vi "Main.vi"(11 "Module Admin":refnum<class "Delacor_lib_QMH_Module Admin.lvclass">) -> ()   [LabVIEW 2019, in "Acquisition.lvlib"]
doc: "This template is based off of the Queued Message Handler design pattern and the Queued Message Handler project template that ships with LabVIEW.\n\nThe main difference is that the queue is private to this module and communication between modules is performed via Broadcast and Request events.\n\nRequest events are wrapped in public API methods and are handled in the Event Handling Loop (EHL) of this VI. Any module can register for Broadcast events sent by this module. The EHL generates messages based on user interface actions.\n\nThe Message Handling Loop (MHL) processes messages generated by the EHL, or by other messages. The messages are string values, so new messages can be added easily to the Message Cases case structure in the MHL. Each message cluster can also provide an optional value for Message Data, which is a variant that can be converted to whatever message-specific data is required.\n_____\nBased on Delacor QMH Project Template 4.0.0.47.\n_____\nBased on DQMH Project Template 6.1.0.94.\n\n<b>Note:</b> This VI was modified by the <b>Validate DQMH Module</b> tool to add a 'Panel Hidden' status updated broadcast to the Panel Close? event when External Launch = TRUE.\n\n<b>Note:</b> This VI was modified by the <b>Validate DQMH Module</b> tool to add a call to the Error Reported VI at the end of the 'Exit' MHL frame."
uses:
  Acquisition.lvlib
  <vilib>/Delacor/Delacor QMH/Libraries/Module Admin_class/Delacor_lib_QMH_Module Admin.lvclass
  Module Data--cluster.ctl
  Signal Type--enum.ctl
  Calibration Values--cluster.ctl
  WiBCI16T_Data.ctl
  WiBCI16T_Status.ctl
  Reg_Map.ctl
  Acquisition Types.ctl
  Stop Argument--cluster.ctl
  <vilib>/Delacor/Delacor QMH/Libraries/Message Queue_class/Delacor_lib_QMH_Message Queue.lvclass/Delacor_lib_QMH_Message Queue.ctl
  <vilib>/Delacor/Delacor QMH/Libraries/Module Admin_class/Delacor_lib_QMH_Module Admin.lvclass/Delacor_lib_QMH_Module Admin.ctl
  Start Acquiring Argument--cluster.ctl
  Start Acquiring (Reply Payload)--cluster.ctl
  Stop Acquiring Argument--cluster.ctl
  Settings Editor/Update Application Settings (Reply Payload)--cluster.ctl
  Settings Editor/Settings--cluster.ctl
  CML Shared/EEG Channel Settings.ctl
  Command_TestData Argument--cluster.ctl
  Check WiFi AP Argument--cluster.ctl
  Command_NoiseData Argument--cluster.ctl
  Command_LiveData Argument--cluster.ctl
  Command_ImpedanceData Argument--cluster.ctl
  Command_GoToIdle Argument--cluster.ctl
  Soft Trigger Argument--cluster.ctl
  Start IMP Acquiring Argument--cluster.ctl
  Stop IMP acquiring Argument--cluster.ctl
  Start GND Loop acquiring Argument--cluster.ctl
  Start CNV Acquiring Argument--cluster.ctl
  Start EOC Acquiring Argument--cluster.ctl
  Command_GndImpedanceData Argument--cluster.ctl
  <vilib>/Utility/miscctls.llb/LVPointTypeDef.ctl
  <vilib>/Delacor/Delacor QMH/Libraries/Message Queue_class/Delacor_lib_QMH_Enqueue Message (Single).vi
  <vilib>/Delacor/Delacor QMH/Libraries/Module Admin_class/Delacor_lib_QMH_Get External Launch.vi
  <userlib>/_MGI/1D Array/MGI Calculate Array Differences/MGI Calculate Array Differences (DBL[]).vi
  <userlib>/_MGI/Timing/MGI Wait/MGI Wait (U32).vi
  <vilib>/Utility/error.llb/Error Cluster From Error Code.vi
  <vilib>/ErrorRing/Error Ring.xnode
  <vilib>/Delacor/Delacor QMH/Libraries/Message Queue_class/Delacor_lib_QMH_Message Queue.lvclass
  Settings Editor/Settings Editor.lvlib
  Logger/Logger.lvlib
  CML UI/CML UI.lvlib
  CML Shared/CML Shared.lvlib
  Lab Streaming Layer/Lab Streaming Layer.lvlib
panel:
  out "Settings":T1 {"WiBCI16T Data"."Reg Map"."ADS2" format="%x"; "WiBCI16T Data"."Reg Map"."ADS1" format="%x"}
  out "error out":errorcluster
  # "This is a headless module. Show its panel to confirm that the Settings are updated correctly and other debugging tasks. Use the Settings Editor to change the settings for this module."
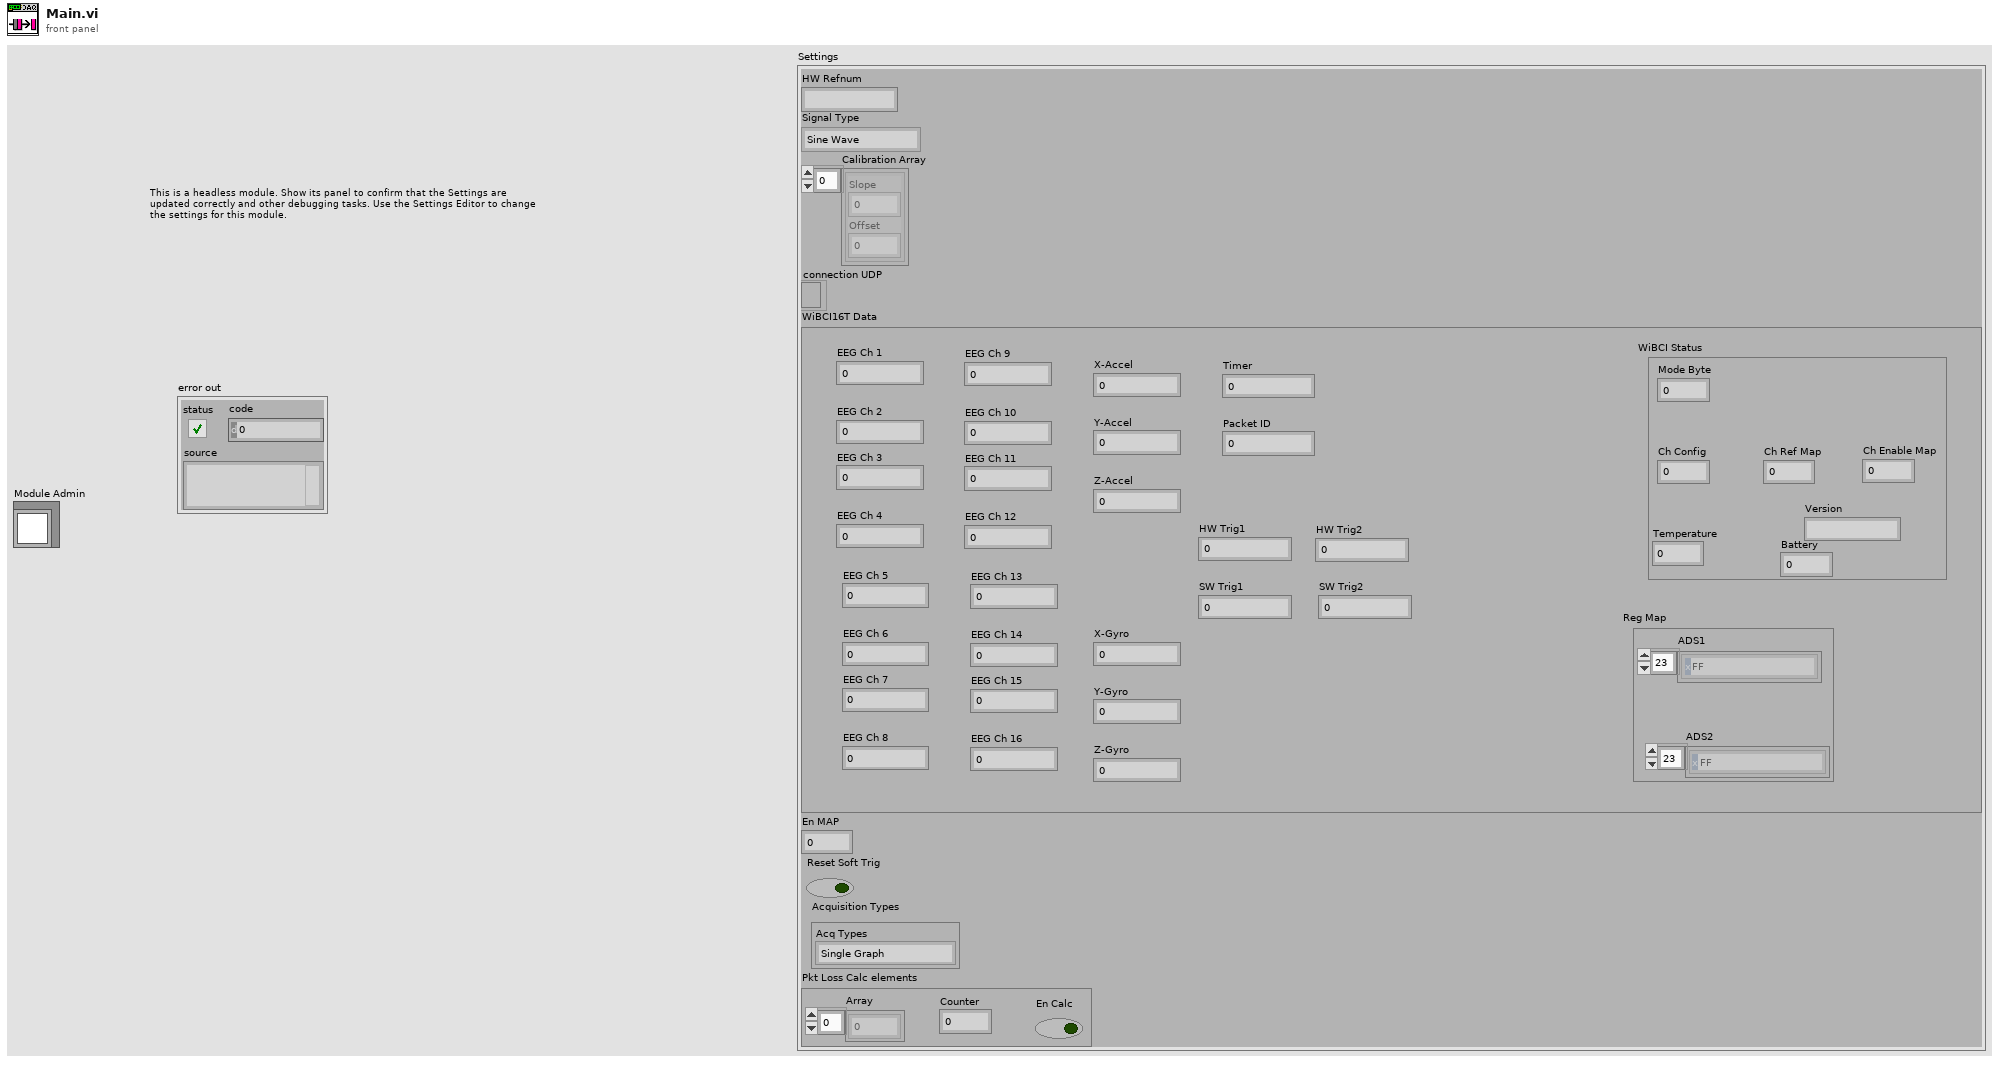
[diagram p1: front panel]
types:
  T1 = typedef "Acquisition.lvlib/Module Data--cluster.ctl" = cluster{"HW Refnum":string, "Signal Type":T2, "Calibration Array":T3[], "connection UDP":refnum<k16>, "WiBCI16T Data":T4, "En MAP":u16, "Reset Soft Trig":bool, "Acquisition Types":T7, "Pkt Loss Calc elements":cluster{"Array":u32[], "Counter":u32, "En Calc":bool}}
  T2 = typedef "Acquisition.lvlib/Signal Type--enum.ctl" = enum16{"Sine Wave", "Square with Noise"}
  T3 = typedef "Acquisition.lvlib/Calibration Values--cluster.ctl" = cluster{"Slope":dbl, "Offset":dbl}
  T4 = typedef "Acquisition.lvlib/WiBCI16T_Data.ctl" = cluster{"EEG Ch 1":dbl, "EEG Ch 2":dbl, "EEG Ch 3":dbl, "EEG Ch 4":dbl, "EEG Ch 5":dbl, "EEG Ch 6":dbl, "EEG Ch 7":dbl, "EEG Ch 8":dbl, "EEG Ch 9":dbl, "EEG Ch 10":dbl, "EEG Ch 11":dbl, "EEG Ch 12":dbl, "EEG Ch 13":dbl, "EEG Ch 14":dbl, "EEG Ch 15":dbl, "EEG Ch 16":dbl, "X-Accel":i16, "Y-Accel":i16, "Z-Accel":i16, "X-Gyro":i16, "Y-Gyro":i16, "Z-Gyro":i16, "Timer":u32, "Packet ID":u32, "HW Trig1":u8, "SW Trig1":i8, "HW Trig2":u8, "SW Trig2":i8, "WiBCI Status":T5, "Reg Map":T6}
  T5 = typedef "Acquisition.lvlib/WiBCI16T_Status.ctl" = cluster{"Mode Byte":u8, "Ch Config":u8, "Ch Ref Map":u16, "Ch Enable Map":u16, "Temperature":sgl, "Battery":u8, "Version":string}
  T6 = typedef "Acquisition.lvlib/Reg_Map.ctl" = cluster{"ADS1":u8[], "ADS2":u8[]}
  T7 = typedef "Acquisition.lvlib/Acquisition Types.ctl" = cluster{"Acq Types":enum16{"Single Graph", "Eyes O/C", "CNV Demo", "Impedance", "Graph"}}
  T8 = typedef "Settings Editor.lvlib/Broadcast Events--cluster.ctl" = cluster{"Module Did Init":refnum<user-event>, "Status Updated":refnum<user-event>, "Error Reported":refnum<user-event>, "Module Did Stop":refnum<user-event>, "Update Module Execution Status":refnum<user-event>, "Application Settings Updated":refnum<user-event>}
  T9 = typedef "Acquisition.lvlib/Request Events--cluster.ctl" = cluster{"Stop Module":refnum<user-event>, "Show Panel":refnum<user-event>, "Hide Panel":refnum<user-event>, "Get Module Execution Status":refnum<user-event>, "Show Diagram":refnum<user-event>, "Stop Acquiring":refnum<user-event>, "Wakeup Helper Loop":refnum<user-event>, "Change Settings":refnum<user-event>, "Calibrate DAQ":refnum<user-event>, "Start Acquiring":refnum<user-event>, "Command_TestData":refnum<user-event>, "Check WiFi AP":refnum<user-event>, "Command_NoiseData":refnum<user-event>, "Command_LiveData":refnum<user-event>, "Command_ImpedanceData":refnum<user-event>, "Command_GoToIdle":refnum<user-event>, "Soft Trigger":refnum<user-event>, "Start IMP Acquiring":refnum<user-event>, "Stop IMP acquiring":refnum<user-event>, "Start GND Loop acquiring":refnum<user-event>, "IMP data updated":refnum<user-event>, "Start CNV Acquiring":refnum<user-event>, "Start EOC Acquiring":refnum<user-event>, "Private":cluster{"Wake-up Helper Loop for Pkt Loss Calc":refnum<user-event>, "Stop Pkt Loss Calc":refnum<user-event>, "Update Packet ID":refnum<user-event>, "Calculate Packet Loss":refnum<user-event>}, "Command_GndImpedanceData":refnum<user-event>}
  T10 = enum32{"invalid lock state", "Not Locked", "Locked (No Password)", "Password-protected"}
  T11 = typedef "Acquisition.lvlib/Stop Argument--cluster.ctl" = cluster{"Origin":string, "Exit via Stop Module Req?":bool, "Wait for Module to stop?":bool}
  T12 = typedef "Acquisition.lvlib/Start Acquiring Argument--cluster.ctl" = cluster{"Wait Notifier":refnum<notifier>, "wait for reply":bool}
  T13 = typedef "Acquisition.lvlib/Stop Acquiring Argument--cluster.ctl" = cluster{"Boolean":bool}
  T14 = typedef "Settings Editor.lvlib/Update Application Settings (Reply Payload)--cluster.ctl" = cluster{"Settings":T15, "error":errorcluster}
  T15 = typedef "Settings Editor.lvlib/Settings--cluster.ctl" = cluster{"Signal Type":T2, "Calibration Array":T3[], "Log File Base Path":path, "EEG Channels":T16, "Soft Trig enum":enum16{"Disable Soft Trigger", "Enable Soft Trigger"}, "Montage selection":cluster{"Montages Ref":refnum<vi>, "Selected Montage Number":u8, "Montages Names":string[]}, "LSL En enum":enum16{"LSL Disabled", "LSL Enabled"}}
  T16 = typedef "CML Shared.lvlib/EEG Channel Settings.ctl" = cluster{"16 EEG Channels":cluster{"Channel Name":string, "Channel No":u8, "Channel Enabled":bool, "Channel Referenced":bool}[], "Gain":u8}
  T17 = typedef "Acquisition.lvlib/Command_TestData Argument--cluster.ctl" = cluster{"Boolean":bool}
  T18 = typedef "Acquisition.lvlib/Check WiFi AP Argument--cluster.ctl" = cluster{"Connected ?":bool}
  T19 = typedef "Acquisition.lvlib/Command_NoiseData Argument--cluster.ctl" = cluster{"Boolean":bool}
  T20 = typedef "Acquisition.lvlib/Command_LiveData Argument--cluster.ctl" = cluster{"Boolean":bool}
  T21 = typedef "Acquisition.lvlib/Command_ImpedanceData Argument--cluster.ctl" = cluster{"Boolean":bool}
  T22 = typedef "Acquisition.lvlib/Command_GoToIdle Argument--cluster.ctl" = cluster{"Boolean":bool}
  T23 = typedef "Acquisition.lvlib/Soft Trigger Argument--cluster.ctl" = cluster{"Value":i8}
  T24 = typedef "Acquisition.lvlib/Start IMP Acquiring Argument--cluster.ctl" = cluster{"Boolean":bool}
  T25 = typedef "Acquisition.lvlib/Stop IMP acquiring Argument--cluster.ctl" = cluster{"Boolean":bool}
  T26 = typedef "Acquisition.lvlib/Start GND Loop acquiring Argument--cluster.ctl" = cluster{"Boolean":bool}
  T27 = typedef "Acquisition.lvlib/Start CNV Acquiring Argument--cluster.ctl" = cluster{"Boolean":bool}
  T28 = typedef "Acquisition.lvlib/Start EOC Acquiring Argument--cluster.ctl" = cluster{"Boolean":bool}
  T29 = typedef "Acquisition.lvlib/Command_GndImpedanceData Argument--cluster.ctl" = cluster{"Boolean":bool}
  T30 = typedef "LVPointTypeDef.ctl" = cluster{"Horizontal":i16, "Vertical":i16}
  T31 = enum32{"Invalid", "Standard", "Closed", "Hidden", "Minimized", "Maximized"}
  T32 = enum16{"Single Graph", "Eyes O/C", "CNV Demo", "Impedance", "Graph"}
  T33 = typedef "Acquisition.lvlib/Start Acquiring (Reply Payload)--cluster.ctl" = cluster{"HW ID":string, "error":errorcluster, "UDP connection ID ":refnum<k16>}
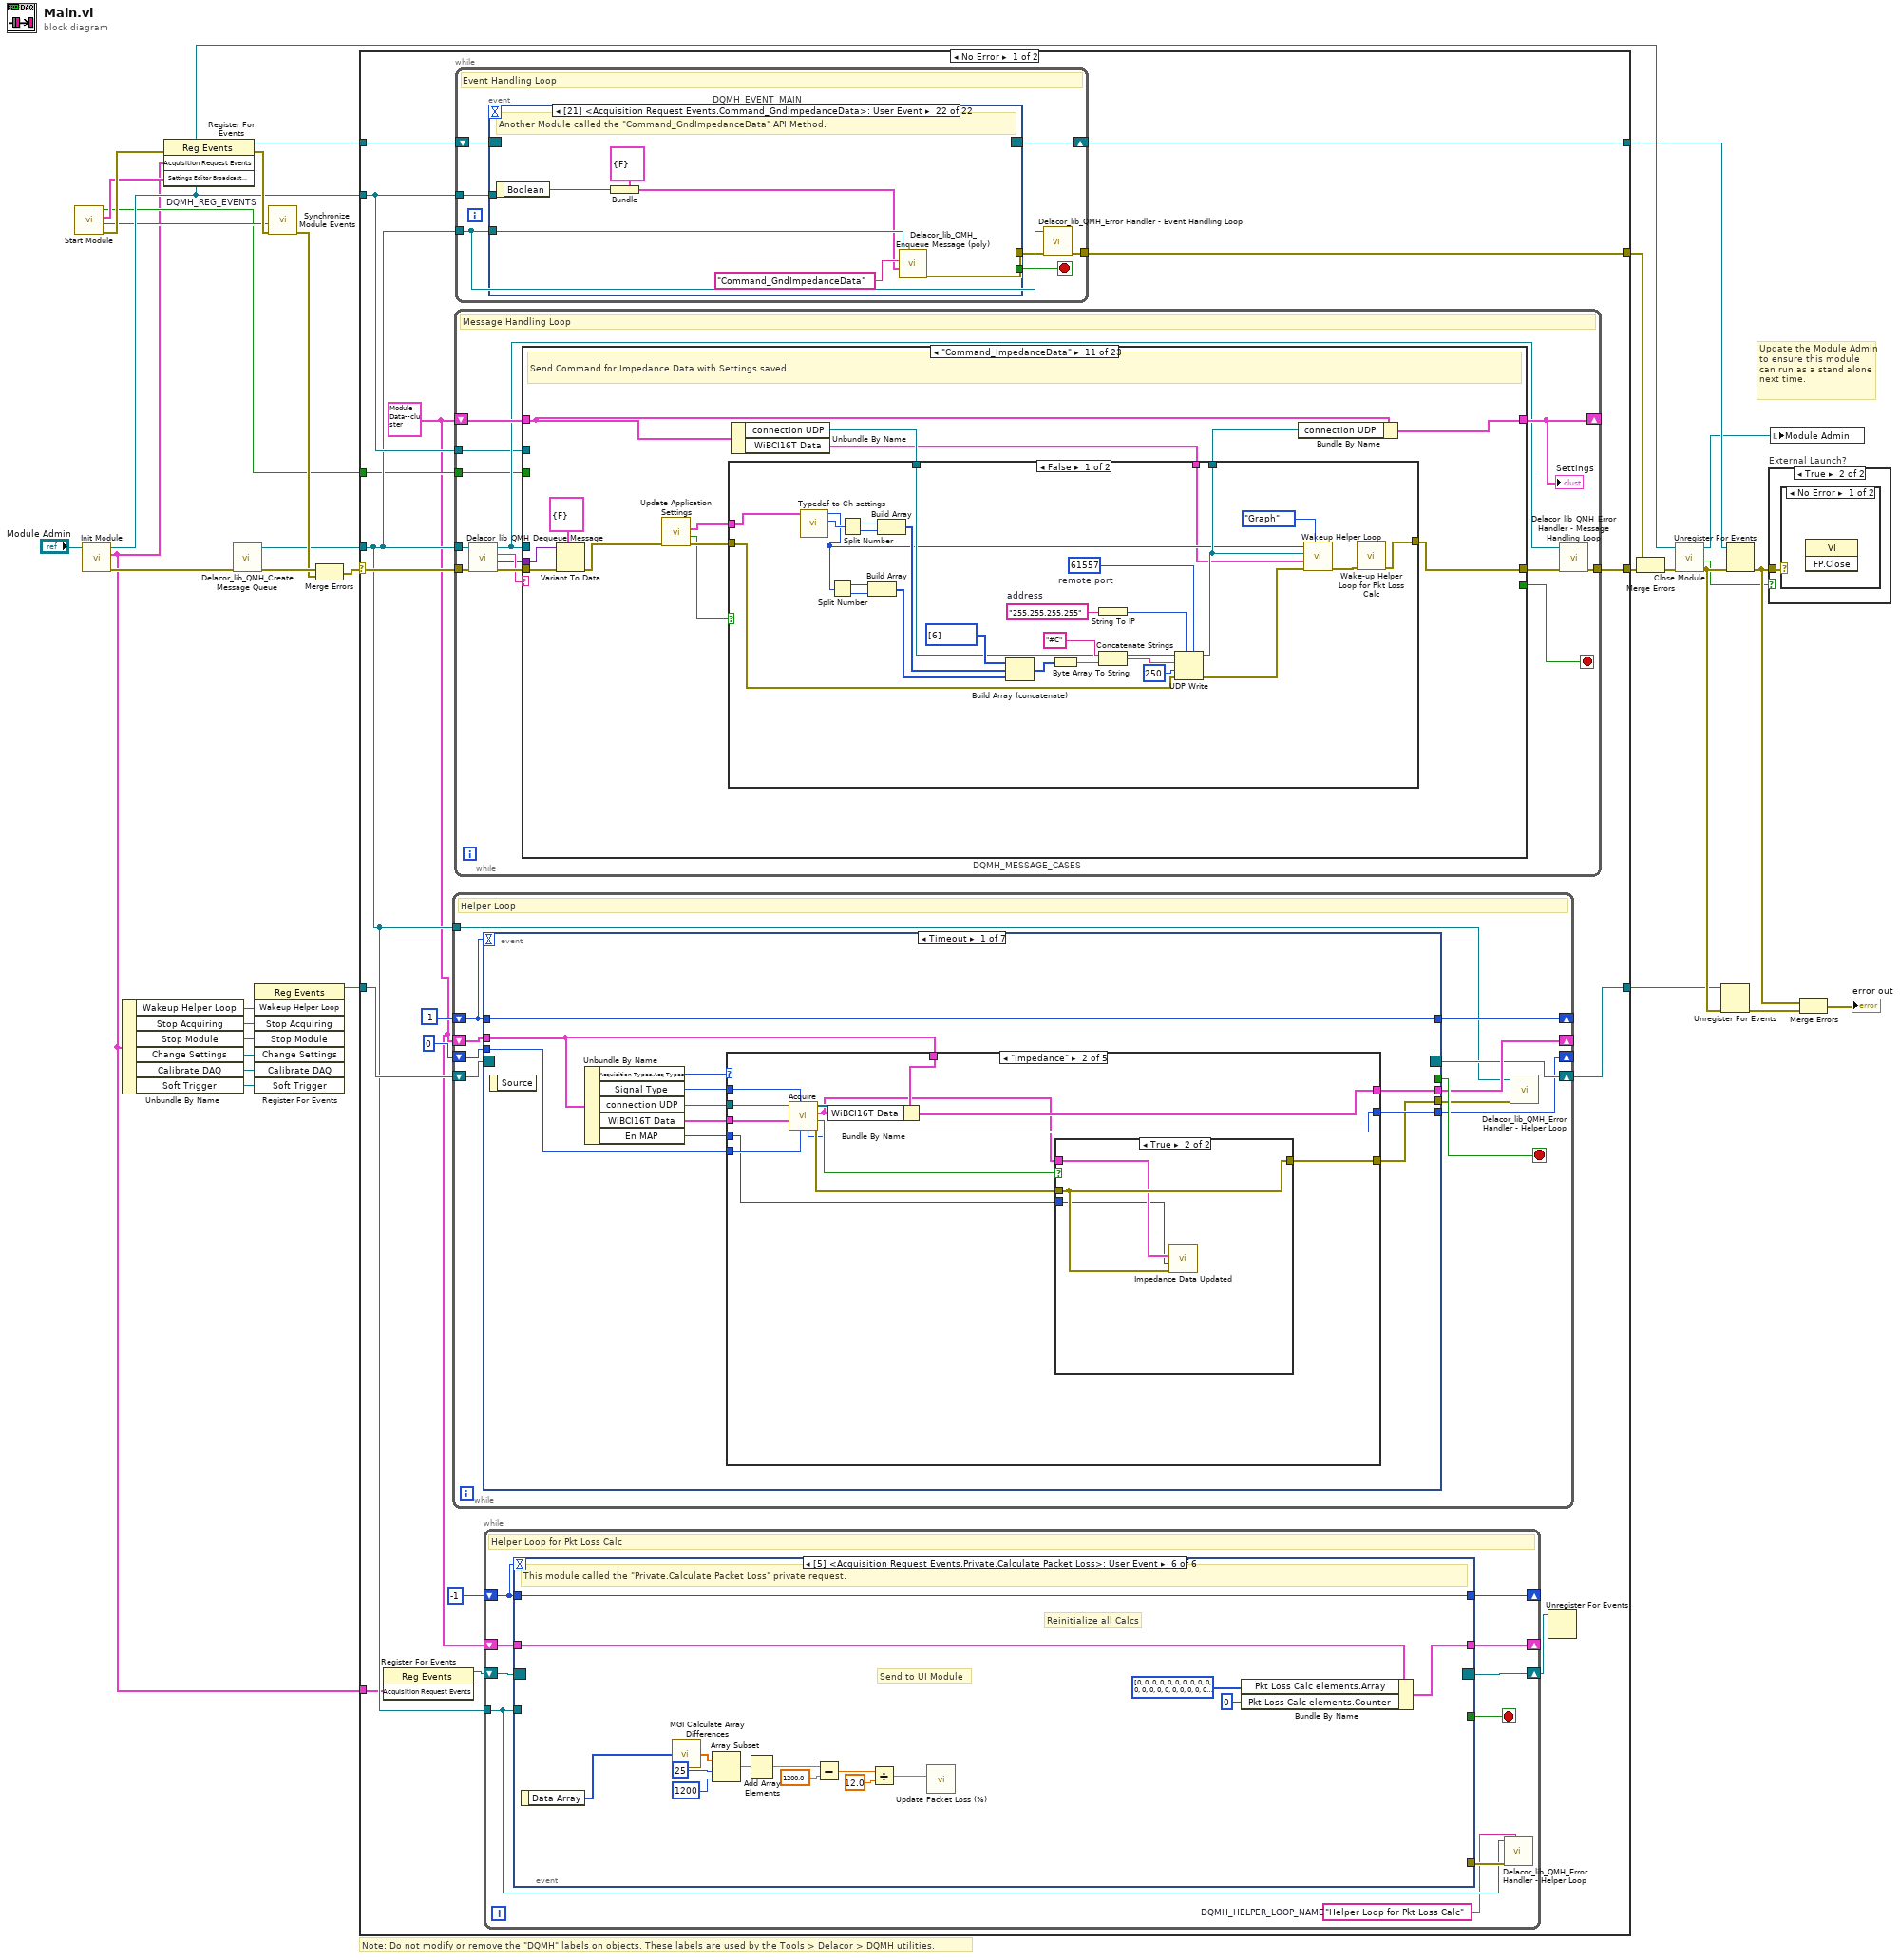
[diagram p0: block diagram]
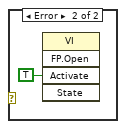
[diagram p3: hidden frame]
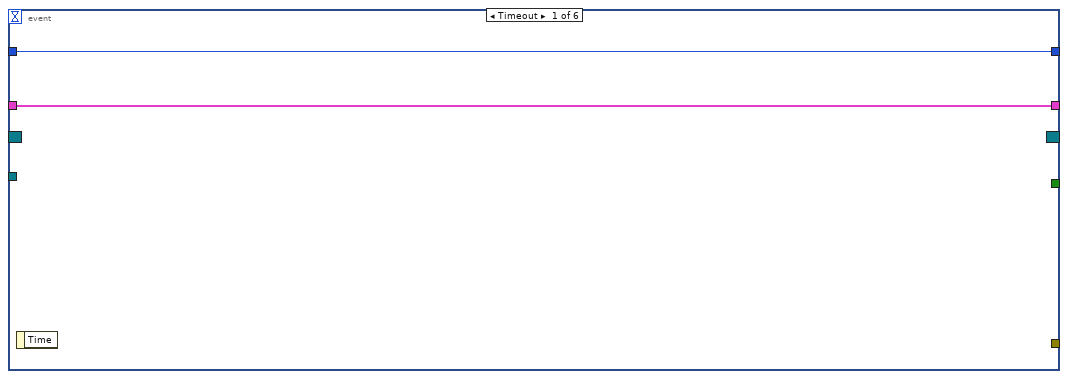
[diagram p4: hidden frame]
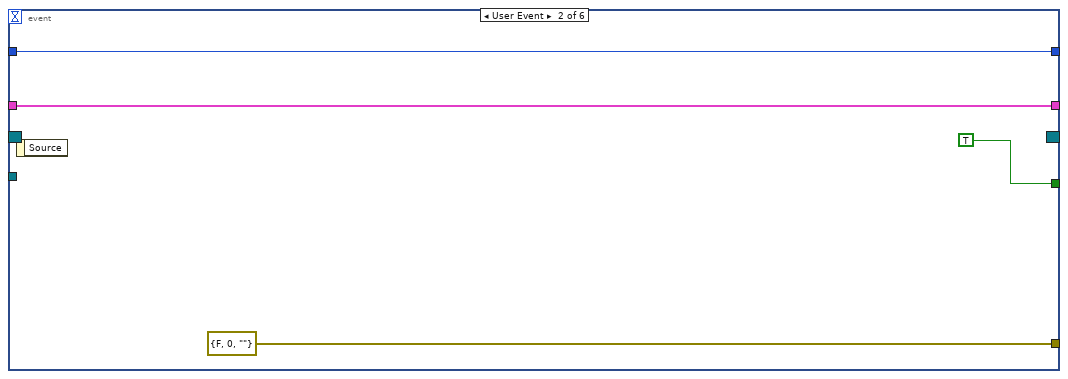
[diagram p5: hidden frame]
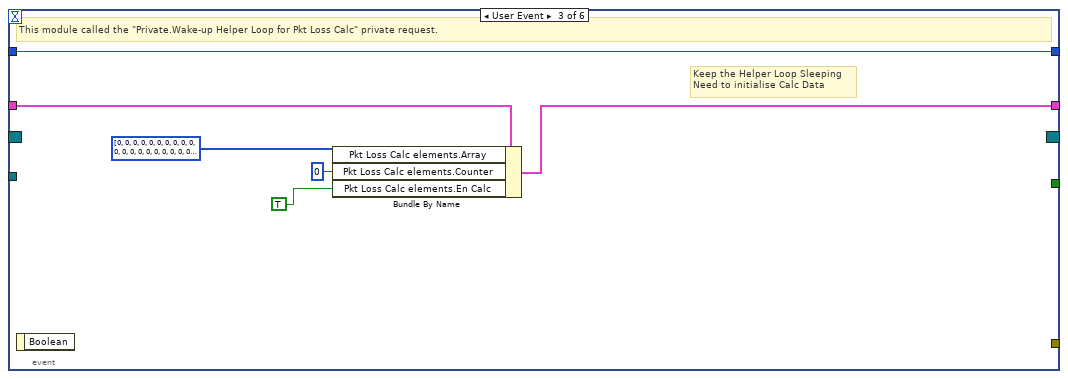
[diagram p6: hidden frame]
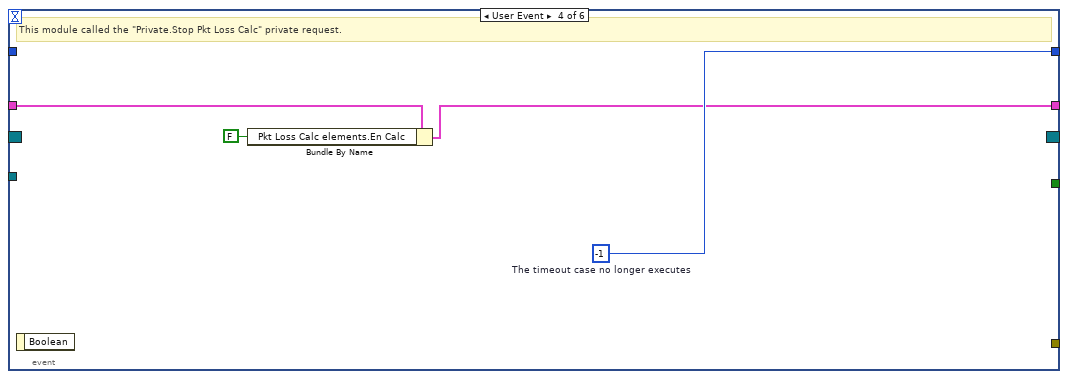
[diagram p7: hidden frame]
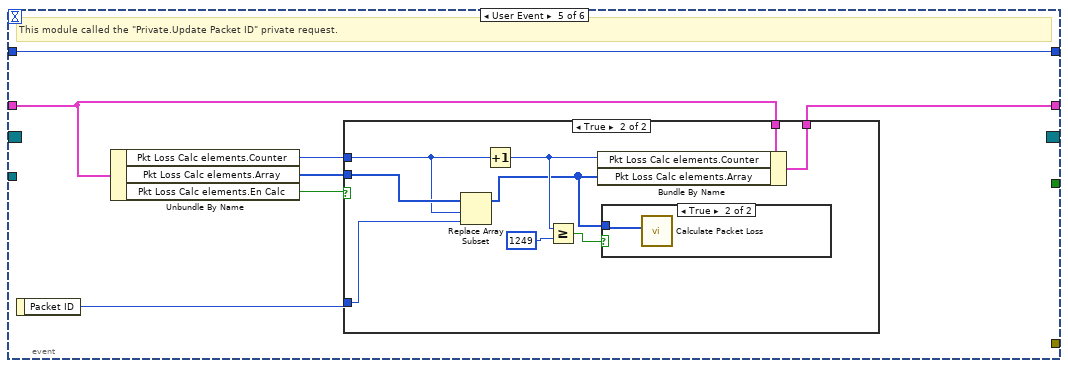
[diagram p8: hidden frame]
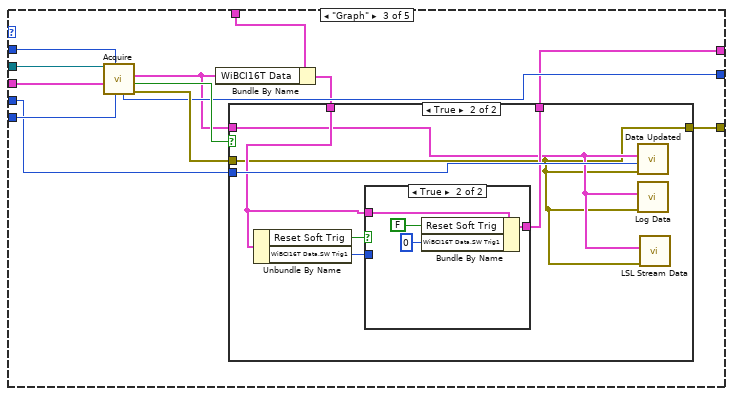
[diagram p13: hidden frame]
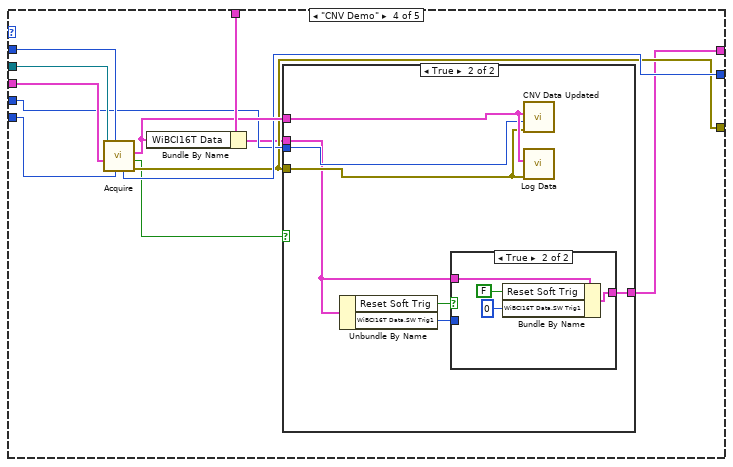
[diagram p16: hidden frame]
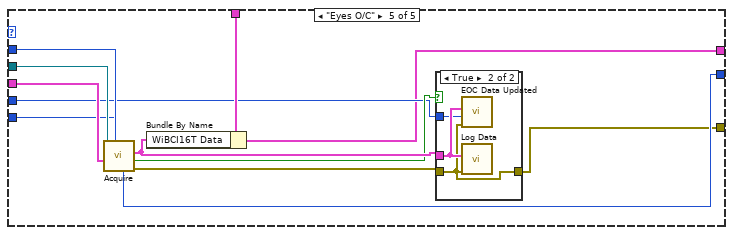
[diagram p19: hidden frame]
diagram:
  # "Note: Do not modify or remove the \"DQMH\" labels on objects. These labels are used by the Tools > Delacor > DQMH utilities."
  # "Update the Module Admin to ensure this module can run as a stand alone next time."
  n1 = call "Start Module.vi"() -> ("error out"=w25:errorcluster, "Wait for Event Sync?"=w7:bool, "Settings Editor Broadcast Events"=w8:T8, "Module Was Already Running?"=w3:bool)  [unwired: 8 in]
  n2 = call "Init Module.vi"("Singleton Module Admin in"="Module Admin") -> ("error out"=w31:errorcluster, "Acquisition Request Events"=w1:T9, "Singleton Module Admin out"=w19:refnum<class "Delacor_lib_QMH_Module Admin.lvclass">)  [unwired: 8 in]
  n3 = Unbundle By Name(w1) -> ("Wakeup Helper Loop"=w9:refnum<user-event>, "Stop Acquiring"=w12:refnum<user-event>, "Stop Module"=w11:refnum<user-event>, "Change Settings"=w6:refnum<user-event>, "Calibrate DAQ"=w5:refnum<user-event>, "Soft Trigger"=w2:refnum<user-event>)
  n4 = register-events "DQMH_REG_EVENTS"(error in=w25, w1, w8) -> (reference out=w17:refnum<event-registration>, error out=w24:errorcluster)  [unwired: 1 in]
  n5 = call <vilib>:"Delacor_lib_QMH_Create Message Queue.vi"("error in"=w31) -> ("error out"=w27:errorcluster, "Message Queue"=w16:refnum<class "Delacor_lib_QMH_Message Queue.lvclass">)  [unwired: 9 in]
  n6 = register-events(w9, w12, w11, w6, w5, w2) -> (reference out=w10:refnum<event-registration>)  [unwired: 2 in, 1 out]
  n7 = call "Synchronize Module Events.vi"("error in (no error)"=w24, "Wait for Event Sync?"=w7) -> ("error out"=w23:errorcluster)  [unwired: 9 in]
  n8 = Merge Errors(w27, w23) -> (w26:errorcluster)
  n9 = case shown="No Error" w26 {
    selector: w26 -> [w47 w928]
    tunnel: [w49 w927] -> w32
    tunnel: [w46 w936] -> w18
    tunnel: w17 -> [w45 w936]
    tunnel: w16 -> [w41 w929]
    tunnel: [w48 _] -> w30
    tunnel: w19 -> [w44 w932]
    tunnel: w10 -> [w42 w931]
    tunnel: [w40 w931] -> w4
    tunnel: w3 -> [w39 w930]
    tunnel: w1 -> [w37 _]
    frame No Error {
      w33 = T1 {"HW Refnum"="", "Signal Type"=enum."Sine Wave", "Calibration Array"=[{"Slope"=1.0, "Offset"=0.0}], "connection UDP"=refnum, "WiBCI16T Data"={"EEG Ch 1"=0.0, "EEG Ch 2"=0.0, "EEG Ch 3"=0.0, "EEG Ch 4"=0.0, "EEG Ch 5"=0.0, "EEG Ch 6"=0.0, "EEG Ch 7"=0.0, "EEG Ch 8"=0.0, "EEG Ch 9"=0.0, "EEG Ch 10"=0.0, "EEG Ch 11"=0.0, "EEG Ch 12"=0.0, "EEG Ch 13"=0.0, "EEG Ch 14"=0.0, "EEG Ch 15"=0.0, "EEG Ch 16"=0.0, "X-Accel"=0, "Y-Accel"=0, "Z-Accel"=0, "X-Gyro"=0, "Y-Gyro"=0, "Z-Gyro"=0, "Timer"=0, "Packet ID"=0, "HW Trig1"=0, "SW Trig1"=0, "HW Trig2"=0, "SW Trig2"=0, "WiBCI Status"={"Mode Byte"=0, "Ch Config"=0, "Ch Ref Map"=0, "Ch Enable Map"=0, "Temperature"=0.0, "Battery"=0, "Version"=""}, "Reg Map"={"ADS1"=[], "ADS2"=[]}}, "En MAP"=0, "Reset Soft Trig"=FALSE, "Acquisition Types"={"Acq Types"=enum."Single Graph"}, "Pkt Loss Calc elements"={"Array"=[], "Counter"=0, "En Calc"=FALSE}} ("Data Cluster")
      n10 = register-events ("DQMH_HELPER_REGFOREVENTS")(w37) -> (reference out=w35:refnum<event-registration>)  [unwired: 2 in, 1 out]
      n11 = while {
        shift-right: [w119] -> _
        shift-left: -1 -> [w118]
        tunnel: w41 -> [w112]
        shift-right: [w115] -> _
        shift-left: w33 -> [w114]
        shift-right: [w113] -> w40
        shift-left: w42 -> [w117]
        shift-right: [w109] -> _
        shift-left: u16 0 -> [w110]
        stop <- w116 stop-if-true
        # "Helper Loop"
        n12 = event shown="[0] Timeout" {
          selector: w117 -> [_ _ _ _ _ _ _]
          dyn-events: [_ _ _ _ _ _ _] -> w113
          timeout: w118 -> [_ _ _ _ _ _ _]
          tunnel: [w130 w222 w232 w236 w246 w249 w257] -> w119
          tunnel: w118 -> [w130 w222 w232 w236 _ _ w257]
          tunnel: [_ _ _ TRUE _ _ _] -> w116
          tunnel: [w122 w223 _ _ _ _ _] -> w111
          tunnel: [w126 w220 w230 w234 w242 w248 w252] -> w115
          tunnel: w114 -> [w120 w221 w231 w234 w244 w248 w253]
          tunnel: w110 -> [w125 w217 w227 w233 w241 w247 w256]
          tunnel: [w124 w217 w227 w233 w241 w247 w256] -> w109
          event Timeout {
            n13 = event-data() -> ()  [unwired: 1 in, 1 out]
            n14 = Unbundle By Name(w120) -> ("Acquisition Types.Acq Types"=w121:T32, "Signal Type"=w129:T2, "connection UDP"=w128:refnum<k16>, "WiBCI16T Data"=w127:T4, "En MAP"=w123:u16)
            n15 = case shown="\"Impedance\"" w121 {
              tunnel: w129 -> [_ w144 w161 w187 w212]
              tunnel: w128 -> [_ w143 w160 w186 w211]
              tunnel: w127 -> [_ w141 w158 w185 w209]
              tunnel: w120 -> [w132 w140 w157 w184 w208]
              tunnel: [w132 w139 w150 w178 w201] -> w126
              tunnel: w125 -> [w131 w137 w155 w182 w205]
              tunnel: [w131 w136 w154 w181 w204] -> w124
              tunnel: w123 -> [_ w135 w153 w180 w203]
              tunnel: [_ w134 w152 w179 w202] -> w122
              frame "Single Graph", Default {
              }
              frame "Impedance" {
                n16 = call "Acquire.vi"("Infm Alive Counter"=w137, "Signal Type"=w144, "WiBCI16T Data"=w141, "connection UDP"=w143) -> ("error out"=w142:errorcluster, "Data Valid ?"=w138:bool, "WiBCI16T Data out"=w133:T4, "Infm Alive Counter out"=w136:u16)  [unwired: 3 in, 1 out]
                n17 = Bundle By Name(cluster=w140, "WiBCI16T Data"=w133) -> (w139:T1)
                n18 = case shown="True" w138 {
                  tunnel: w142 -> [w145 w148]
                  tunnel: w133 -> [_ w147]
                  tunnel: w135 -> [_ w146]
                  tunnel: [w145 w148] -> w134
                  frame False {
                  }
                  frame True {
                    n19 = call "Impedance Data Updated.vi"("error in"=w148, "En MAP"=w146, "WiBCI16T Data"=w147) -> ()  [unwired: 8 in, 1 out]
                  }
                }
              }
              frame "Graph" {
                n20 = call "Acquire.vi"("Infm Alive Counter"=w155, "Signal Type"=w161, "WiBCI16T Data"=w158, "connection UDP"=w160) -> ("error out"=w159:errorcluster, "Data Valid ?"=w156:bool, "WiBCI16T Data out"=w149:T4, "Infm Alive Counter out"=w154:u16)  [unwired: 3 in, 1 out]
                n21 = Bundle By Name(cluster=w157, "WiBCI16T Data"=w149) -> (w151:T1)
                n22 = case shown="True" w156 {
                  tunnel: w159 -> [w163 w164]
                  tunnel: w149 -> [_ w165]
                  tunnel: w153 -> [_ w170]
                  tunnel: [w163 w164] -> w152
                  tunnel: w151 -> [w162 w168]
                  tunnel: [w162 w167] -> w150
                  frame False {
                  }
                  frame True {
                    n23 = Unbundle By Name(w168) -> ("Reset Soft Trig"=w169:bool, "WiBCI16T Data.SW Trig1"=w166:i8)
                    n24 = case shown="True" w169 {
                      tunnel: w168 -> [w171 w175]
                      tunnel: [w171 w173] -> w167
                      tunnel: w166 -> [_ _]
                      frame False {
                      }
                      frame True {
                        n25 = Bundle By Name(cluster=w175, "Reset Soft Trig"=FALSE, "WiBCI16T Data.SW Trig1"=i8 0) -> (w173:T1)
                      }
                    }
                    n26 = call "Data Updated.vi"("error in (no error)"=w164, "En MAP"=w170, "WiBCI16T Data in"=w165) -> ()  [unwired: 8 in, 1 out]
                    n27 = call "Log Data.vi"("error in (no error)"=w164, "WiBCI16T Data out"=w165) -> ()  [unwired: 9 in, 1 out]
                    n28 = call "LSL Stream Data.vi"("error in"=w164, "WiBCI16T Data"=w165) -> ()  [unwired: 9 in, 1 out]
                  }
                }
              }
              frame "CNV Demo" {
                n29 = call "Acquire.vi"("Infm Alive Counter"=w182, "Signal Type"=w187, "WiBCI16T Data"=w185, "connection UDP"=w186) -> ("error out"=w179:errorcluster, "Data Valid ?"=w176:bool, "WiBCI16T Data out"=w183:T4, "Infm Alive Counter out"=w181:u16)  [unwired: 3 in, 1 out]
                n30 = Bundle By Name(cluster=w184, "WiBCI16T Data"=w183) -> (w177:T1)
                n31 = case shown="True" w176 {
                  tunnel: w183 -> [_ w195]
                  tunnel: w180 -> [_ w194]
                  tunnel: w179 -> [_ w193]
                  tunnel: [w188 w190] -> w178
                  tunnel: w177 -> [w188 w189]
                  frame False {
                  }
                  frame True {
                    n32 = Unbundle By Name(w189) -> ("Reset Soft Trig"=w192:bool, "WiBCI16T Data.SW Trig1"=w191:i8)
                    n33 = case shown="True" w192 {
                      tunnel: w189 -> [w196 w200]
                      tunnel: [w196 w198] -> w190
                      tunnel: w191 -> [_ _]
                      frame False {
                      }
                      frame True {
                        n34 = Bundle By Name(cluster=w200, "Reset Soft Trig"=FALSE, "WiBCI16T Data.SW Trig1"=i8 0) -> (w198:T1)
                      }
                    }
                    n35 = call "CNV Data Updated.vi"("error in"=w193, "En MAP"=w194, "WiBCI16T Data"=w195) -> ()  [unwired: 8 in, 1 out]
                    n36 = call "Log Data.vi"("error in (no error)"=w193, "WiBCI16T Data out"=w195) -> ()  [unwired: 9 in, 1 out]
                  }
                }
              }
              frame "Eyes O/C" {
                n37 = call "Acquire.vi"("Infm Alive Counter"=w205, "Signal Type"=w212, "WiBCI16T Data"=w209, "connection UDP"=w211) -> ("error out"=w210:errorcluster, "Data Valid ?"=w206:bool, "WiBCI16T Data out"=w207:T4, "Infm Alive Counter out"=w204:u16)  [unwired: 3 in, 1 out]
                n38 = Bundle By Name(cluster=w208, "WiBCI16T Data"=w207) -> (w201:T1)
                n39 = case shown="True" w206 {
                  tunnel: w210 -> [w213 w214]
                  tunnel: w207 -> [_ w216]
                  tunnel: w203 -> [_ w215]
                  tunnel: [w213 w214] -> w202
                  frame False {
                  }
                  frame True {
                    n40 = call "EOC Data Updated.vi"("error in"=w214, "En MAP"=w215, "WiBCI16T Data"=w216) -> ()  [unwired: 8 in, 1 out]
                    n41 = call "Log Data.vi"("error in (no error)"=w214, "WiBCI16T Data out"=w216) -> ()  [unwired: 9 in, 1 out]
                  }
                }
              }
            }
          }
          event User Event {
            n42 = event-data() -> ()  [unwired: 1 in, 1 out]
            n43 = in-place {
              in-place-border: [w226] -> w219
              n44 = in-place-cluster #1(w221) -> ("Calibration Array"=w225:T3[])
              n45 = call "Calibration Routine State Machine.vi"("Calibration Array in"=w225) -> ("error out"=w226:errorcluster, "Calibration Array out"=w224:T3[])  [unwired: 9 in]
              n46 = in-place-cluster #1("Calibration Array"=w224) -> (w220:T1)
            }
            n47 = call "Status Updated.vi"("error in (no error)"=w219, "Status"="Device successfully calibrated") -> ()  [unwired: 9 in, 1 out]
            n48 = call "Device Calibrated.vi"("error in (no error)"=w219) -> ("error out"=w223:errorcluster)  [unwired: 10 in]
          }
          event User Event {
            n49 = event-data() -> ("Signal Type"=w229:T2, "Calibration Array"=w228:T3[])  [unwired: 1 in]
            n50 = Bundle By Name(cluster=w231, "Signal Type"=w229, "Calibration Array"=w228) -> (w230:T1)
          }
          event User Event {
            n51 = event-data() -> ()  [unwired: 1 in, 1 out]
          }
          event User Event {
            w246 = 0  # Change the timeout to ensure the timeout case executes
            n52 = event-data() -> ("En MAP"=w240:u16, "connection UDP"=w243:refnum<k16>, "Acquisition Types.Acq Types"=w239:T32)  [unwired: 1 in]
            n53 = Bundle By Name(cluster=w244, "connection UDP"=w243, "En MAP"=w240, "Acquisition Types.Acq Types"=w239, "Reset Soft Trig"=FALSE, "WiBCI16T Data.SW Trig1"=i8 0) -> (w242:T1)
            n54 = call "Status Updated.vi"("Status"="Acquiring Data ...") -> ()  [unwired: 10 in, 1 out]
          }
          event User Event {
            w249 = -1  # The timeout case no longer executes
            n55 = event-data() -> ()  [unwired: 1 in, 1 out]
          }
          event User Event {
            n56 = event-data() -> ("Value"=w254:i8)  [unwired: 1 in, 4 out]
            n57 = Unbundle By Name(w253) -> ("WiBCI16T Data.SW Trig1"=w255:i8)
            n58 = Add(x=w255, y=w254) -> (x+y=w251:i8)
            n59 = Bundle By Name(cluster=w253, "WiBCI16T Data.SW Trig1"=w251, "Reset Soft Trig"=TRUE) -> (w252:T1)
          }
        }
        n60 = call-dynamic "Delacor_lib_QMH_Error Handler - Helper Loop.vi"("error in"=w111, "Message Queue in"=w112) -> ()  [unwired: 8 in, 2 out]
      }
      n61 = while {
        tunnel: w41 -> [w403]
        shift-right: [w407] -> _
        shift-left: w33 -> [w408]
        tunnel: w47 -> [w411]
        tunnel: [w409] -> w49
        tunnel: w44 -> [w401]
        tunnel: w39 -> [w400]
        stop <- w406 stop-if-true
        # "Message Handling Loop"
        n62 = call-dynamic "Delacor_lib_QMH_Dequeue Message.vi"("error in"=w411, "Message Queue in"=w403) -> ("error out"=w410:errorcluster, "Message Data"=w404:variant, "Message"=w405:string, "Message Queue out"=w402:refnum<class "Delacor_lib_QMH_Message Queue.lvclass">)  [unwired: 6 in]
        n63 = case "DQMH_MESSAGE_CASES" shown="\"Command_ImpedanceData\"" w405 {
          selector: w405 -> [_ _ _ _ _ _ _ _ _ _ _ _ _ _ _ _ _ _ _ _ _ _ w914]
          tunnel: w402 -> [_ _ _ _ _ _ _ _ _ _ _ _ _ _ _ _ _ _ _ _ w879 w903 _]
          tunnel: w410 -> [w433 w443 w467 w475 w485 w507 w529 w542 w584 w625 w666 w707 w748 w796 w802 w807 w813 w816 w823 w876 w886 w910 w917]
          tunnel: [w414 w443 w466 w473 w477 w486 w508 w535 w578 w619 w656 w698 w739 w777 w798 w805 w811 w815 w827 w876 w882 w907 w918] -> w412
          tunnel: w408 -> [w422 w442 w459 w470 w482 w493 w514 w537 w580 w621 w658 w700 w741 w780 w801 w806 w812 w814 w829 w875 w881 w895 w915]
          tunnel: [w417 w442 w459 w470 w482 w491 w513 w536 w579 w620 w657 w699 w740 w781 w801 w806 w812 w814 w828 w875 w881 w895 w915] -> w407
          tunnel: [_ _ _ _ _ _ _ _ _ _ _ _ _ _ _ _ _ _ _ _ _ w902 _] -> w406
          tunnel: w404 -> [_ _ w465 w472 w483 w506 w528 w541 w583 w624 w665 w706 w747 w795 w800 w804 w810 _ w824 _ w880 w901 _]
          tunnel: w401 -> [w423 _ _ _ _ _ _ _ _ _ _ _ _ _ _ _ _ _ _ _ w878 w896 _]
          tunnel: w400 -> [_ _ _ _ _ _ _ _ _ _ _ _ _ _ _ _ _ _ _ _ _ w894 _]
          frame "Initialize" {
            # "Initialize - Any operation that needs to be done before the module can receive messages. Synchronize Caller Events.vi will inform Start Module.vi that the module has launched and is ready to receive messages. Module Did Init.vi will broadcast that the module initialized."
            n64 = call "Synchronize Caller Events.vi"("error in (no error)"=w433, "Singleton Module Admin in"=w423) -> ("error out"=w432:errorcluster, "Singleton Module Admin out"=w419:refnum<class "Delacor_lib_QMH_Module Admin.lvclass">)  [unwired: 8 in]
            n65 = call "Update Application Settings.vi"("wait for reply (T)"=TRUE) -> ("timed out?"=w413:bool, "Reply Payload"=w416:T14)  [unwired: 8 in, 1 out]
            n66 = property class="Module Admin"(reference=w419) -> ("Accessors:External Launch"=w427:bool)  [unwired: 1 in, 2 out]
            n67 = case shown="True" w413 {
              tunnel: w422 -> [w440 w441]
              tunnel: [w439 w441] -> w417
              tunnel: w416 -> [w438 _]
              frame False {
                n68 = Unbundle By Name(w438) -> ("Settings.Signal Type"=w437:T2, "Settings.Calibration Array"=w436:T3[])
                n69 = Bundle By Name(cluster=w440, "Signal Type"=w437, "Calibration Array"=w436) -> (w439:T1)
              }
              frame True {
              }
            }
            n70 = Select(t=T31."Hidden" ("State"), s=w427, f=T31."Standard" ("State")) -> (s? t:f=w424:T31)
            n71 = call "Module Name--constant.vi"() -> ("Module Name"=w430:string)  [unwired: 11 in]
            n72 = property class="VI"("Front Panel.Title"=w430) -> (reference out=w429:refnum<vi>, error out=w435:errorcluster)  [unwired: 2 in]
            n73 = call "Module Name--constant.vi"() -> ("Module Name"=w420:string)  [unwired: 11 in]
            n74 = invoke class="VI" method="FP.Open"(reference=w429, error in=w435, "State"=w424) -> (reference out=w428:refnum<vi>, error out=w434:errorcluster)  [unwired: 2 in, 3 out]
            n75 = call "Module Did Init.vi"("error in (no error)"=w432, "Initialized?"=TRUE, "Origin"=w420) -> ("error out"=w431:errorcluster)  [unwired: 8 in]
            n76 = invoke class="VI" method="FP.Center"(reference=w428, error in=w434) -> ()  [unwired: 1 in, 3 out]
            n77 = Merge Errors(w431) -> (w414:errorcluster)
            n78 = property on="Pane" class="Pane"("Origin"=T30 {"Horizontal"=0, "Vertical"=0}) -> ()  [unwired: 2 in, 2 out]
          }
          frame "---Module Specific---" {
            # "Separator -- The following cases handle messages specific to this Module."
          }
          frame "Start Acquiring" {
            w453 = "255.255.255.255"  # address
            w454 = u16 61557  # remote port
            # "Requests Acquisition Module to start acquiring."
            n79 = Variant To Data(error in=w467, type=T12 {"Wait Notifier"=refnum, "wait for reply"=FALSE} ("Start Acquisition Argument"), Variant=w465) -> (data=w463:T12, error out=w451:errorcluster)
            n80 = Unbundle By Name(w459) -> ("connection UDP"=w450:refnum<k16>, "WiBCI16T Data"=w445:T4)
            n81 = Byte Array To String(unsigned byte array=u8[] [4, 0, 0, 0, 0]) -> (string=w458:string)
            n82 = String To IP(1:w453) -> (0:w452:u32)
            n83 = Concatenate Strings("#C", w458) -> (w455:string)
            n84 = UDP Write(address=w452, port or service name=w454, connection ID=w450, data in=w455, 8:w451, 9:250 ("timeout ms (25000)")) -> (error out=w449:errorcluster, 3:w448:refnum<k16>)
            n85 = Unbundle By Name(w463) -> ("Wait Notifier"=w462:refnum<notifier>)
            n86 = Bundle By Name(cluster=T33 {"HW ID"="", "error"={"status"=FALSE, "code"=0, "source"=""}, "UDP connection ID "=refnum} ("Start Acquisition (Reply Payload)"), "UDP connection ID"=w448, "error"=w449) -> (w461:T33)
            n87 = call "Wakeup Helper Loop.vi"("Acquisition Types.Acq Types"=T32."Graph", "error in (no error)"=w449, "WiBCI16T Data out"=w445, "connection UDP"=w448, "En MAP"=u16 65535) -> ("error out"=w466:errorcluster)  [unwired: 6 in]
            n88 = Send Notification(notification=w461, notifier=w462) -> ()  [unwired: 1 in, 2 out]
          }
          frame "Stop Acquiring" {
            # "Requests the Acquisition Module to stop acquiring"
            n89 = Variant To Data(error in=w475, type=T13 {"Boolean"=FALSE} ("Stop Acquiring Argument"), Variant=w472) -> (error out=w474:errorcluster)  [unwired: 1 out]
            n90 = Unbundle By Name(w470) -> ("HW Refnum"=w469:string)
            n91 = call "Stop Acquisition.vi"("error in (no error)"=w474, "HW Refnum"=w469) -> ("error out"=w473:errorcluster)  [unwired: 9 in]
            n92 = call "Acquisition Stopped.vi"("error in (no error)"=w473) -> ()  [unwired: 10 in, 1 out]
            n93 = call "Status Updated.vi"("error in (no error)"=w473, "Status"="Acquisition Stopped") -> ()  [unwired: 9 in, 1 out]
          }
          frame "Update Settings" {
            # "Send the Change Settings event to the helper loop."
            # "The Settings Editor broadcasted that the settings have changed."
            n94 = Variant To Data(error in=w485, type=T14 {"Settings"={"Signal Type"=enum."Sine Wave", "Calibration Array"=[], "Log File Base Path"=path "", "EEG Channels"={"16 EEG Channels"=[], "Gain"=24}, "Soft Trig enum"=enum."Disable Soft Trigger", "Montage selection"={"Montages Ref"=refnum, "Selected Montage Number"=0, "Montages Names"=[]}, "LSL En enum"=enum."LSL Disabled"}, "error"={"status"=FALSE, "code"=0, "source"=""}} ("Settings Updated Argument"), Variant=w483) -> (data=w480:T14, error out=w484:errorcluster)
            n95 = Unbundle By Name(w480) -> ("Settings.Signal Type"=w479:T2, "Settings.Calibration Array"=w478:T3[])
            n96 = call "Change Settings.vi"("error in (no error)"=w484, "Calibration Array"=w478, "Signal Type"=w479) -> ("error out"=w477:errorcluster)  [unwired: 8 in]
            n97 = call "Status Updated.vi"("error in (no error)"=w477, "Status"="Settings Updated") -> ()  [unwired: 9 in, 1 out]
          }
          frame "Command_TestData" {
            w499 = "255.255.255.255"  # address
            w500 = u16 61557  # remote port
            # "Comand for Test Data as per API 2.4"
            n98 = Variant To Data(error in=w507, type=T17 {"Boolean"=FALSE} ("Command_TestData Argument"), Variant=w506) -> (error out=w492:errorcluster)  [unwired: 1 out]
            n99 = Unbundle By Name(w493) -> ("connection UDP"=w497:refnum<k16>, "WiBCI16T Data"=w489:T4)
            n100 = Byte Array To String(unsigned byte array=u8[] [4, 0, 0, 0, 0]) -> (string=w504:string)
            n101 = String To IP(1:w499) -> (0:w498:u32)
            n102 = Concatenate Strings("#C", w504) -> (w501:string)
            n103 = UDP Write(address=w498, port or service name=w500, connection ID=w497, data in=w501, 8:w492, 9:250 ("timeout ms (25000)")) -> (error out=w496:errorcluster, 3:w495:refnum<k16>)
            n104 = Bundle By Name(cluster=w493, "connection UDP"=w495) -> (w491:T1)
            n105 = call "Wakeup Helper Loop.vi"("Acquisition Types.Acq Types"=T32."Graph", "error in (no error)"=w496, "WiBCI16T Data out"=w489, "connection UDP"=w495, "En MAP"=u16 65535) -> ("error out"=w487:errorcluster)  [unwired: 6 in]
            n106 = call "Wake-up Helper Loop for Pkt Loss Calc.vi"("error in"=w487) -> ("error out"=w486:errorcluster)  [unwired: 10 in]
          }
          frame "Command_NoiseData" {
            w521 = "255.255.255.255"  # address
            w522 = u16 61557  # remote port
            # "Send Noise Data Command as per API 2.4"
            n107 = Variant To Data(error in=w529, type=T19 {"Boolean"=FALSE} ("Command_NoiseData Argument"), Variant=w528) -> (error out=w515:errorcluster)  [unwired: 1 out]
            n108 = Unbundle By Name(w514) -> ("connection UDP"=w519:refnum<k16>, "WiBCI16T Data"=w511:T4)
            n109 = Byte Array To String(unsigned byte array=u8[] [5, 0, 0, 0, 0]) -> (string=w526:string)
            n110 = String To IP(1:w521) -> (0:w520:u32)
            n111 = Concatenate Strings("#C", w526) -> (w523:string)
            n112 = UDP Write(address=w520, port or service name=w522, connection ID=w519, data in=w523, 8:w515, 9:250 ("timeout ms (25000)")) -> (error out=w518:errorcluster, 3:w517:refnum<k16>)
            n113 = Bundle By Name(cluster=w514, "connection UDP"=w517) -> (w513:T1)
            n114 = call "Wakeup Helper Loop.vi"("Acquisition Types.Acq Types"=T32."Graph", "error in (no error)"=w518, "WiBCI16T Data out"=w511, "connection UDP"=w517, "En MAP"=u16 65535) -> ("error out"=w509:errorcluster)  [unwired: 6 in]
            n115 = call "Wake-up Helper Loop for Pkt Loss Calc.vi"("error in"=w509) -> ("error out"=w508:errorcluster)  [unwired: 10 in]
          }
          frame "Command_LiveData" {
            # "Acquire Live Data as per the settings saved in configuration"
            n116 = Variant To Data(error in=w542, type=T20 {"Boolean"=FALSE} ("Command_LiveData Argument"), Variant=w541) -> (error out=w534:errorcluster)  [unwired: 1 out]
            n117 = call "Update Application Settings.vi"("error in"=w534) -> ("error out"=w533:errorcluster, "timed out?"=w532:bool, "Reply Payload"=w531:T14)  [unwired: 8 in]
            n118 = Unbundle By Name(w537) -> ("connection UDP"=w539:refnum<k16>, "WiBCI16T Data"=w530:T4)
            n119 = case shown="False" w532 {
              tunnel: w539 -> [w559 w571]
              tunnel: [w558 w571] -> w538
              tunnel: [w543 w569] -> w535
              tunnel: w533 -> [w557 w570]
              tunnel: w531 -> [w556 _]
              tunnel: w530 -> [w546 _]
              frame False {
                w563 = "255.255.255.255"  # address
                w564 = u16 61557  # remote port
                n120 = call "Typedef to Ch settings.vi"("Reply Payload"=w556) -> ("Referenced Channels"=w554:u16, "Enabled Channels"=w547:u16)  [unwired: 9 in]
                n121 = Split Number(x=w547) -> (hi(x)=w549:u8, lo(x)=w550:u8)
                n122 = Split Number(x=w554) -> (hi(x)=w553:u8, lo(x)=w552:u8)
                n123 = Build Array(w549, w550) -> (w548:u8[])
                n124 = Build Array(w553, w552) -> (w551:u8[])
                n125 = Build Array (concatenate)(u8[] [3] ("unsigned byte array"), w551, w548) -> (w555:u8[])
                n126 = Byte Array To String(unsigned byte array=w555) -> (string=w568:string)
                n127 = String To IP(1:w563) -> (0:w562:u32)
                n128 = Concatenate Strings("#C", w568) -> (w565:string)
                n129 = UDP Write(address=w562, port or service name=w564, connection ID=w559, data in=w565, 8:w557, 9:250 ("timeout ms (25000)")) -> (error out=w561:errorcluster, 3:w558:refnum<k16>)
                n130 = call "Wakeup Helper Loop.vi"("Acquisition Types.Acq Types"=T32."Graph", "error in (no error)"=w561, "WiBCI16T Data out"=w546, "connection UDP"=w558, "En MAP"=w547) -> ("error out"=w544:errorcluster)  [unwired: 6 in]
                n131 = call "Wake-up Helper Loop for Pkt Loss Calc.vi"("error in"=w544) -> ("error out"=w543:errorcluster)  [unwired: 10 in]
              }
              frame True {
                n132 = call <vilib>:"Clear Errors.vi"("error in (no error)"=w570) -> ("error out"=w569:errorcluster)  [unwired: 5 in, 1 out]
              }
            }
            n133 = Bundle By Name(cluster=w537, "connection UDP"=w538) -> (w536:T1)
          }
          frame "Start CNV Acquiring" {
            # "Acquire CNV Live Data"
            n134 = Variant To Data(error in=w584, type=T27 {"Boolean"=FALSE} ("Start CNV Acquiring Argument"), Variant=w583) -> (error out=w577:errorcluster)  [unwired: 1 out]
            n135 = call "Update Application Settings.vi"("error in"=w577) -> ("error out"=w576:errorcluster, "timed out?"=w575:bool, "Reply Payload"=w574:T14)  [unwired: 8 in]
            n136 = Unbundle By Name(w580) -> ("connection UDP"=w582:refnum<k16>, "WiBCI16T Data"=w573:T4)
            n137 = case shown="True" w575 {
              tunnel: w582 -> [w600 w612]
              tunnel: [w599 w612] -> w581
              tunnel: [w598 w610] -> w578
              tunnel: w576 -> [w597 w611]
              tunnel: w574 -> [w596 _]
              tunnel: w573 -> [w586 _]
              frame False {
                w604 = "255.255.255.255"  # address
                w605 = u16 61557  # remote port
                n138 = call "Typedef to Ch settings.vi"("Reply Payload"=w596) -> ("Referenced Channels"=w594:u16, "Enabled Channels"=w587:u16)  [unwired: 9 in]
                n139 = Split Number(x=w587) -> (hi(x)=w589:u8, lo(x)=w590:u8)
                n140 = Split Number(x=w594) -> (hi(x)=w593:u8, lo(x)=w592:u8)
                n141 = Build Array(w589, w590) -> (w588:u8[])
                n142 = Build Array(w593, w592) -> (w591:u8[])
                n143 = Build Array (concatenate)(u8[] [3] ("unsigned byte array"), w591, w588) -> (w595:u8[])
                n144 = Byte Array To String(unsigned byte array=w595) -> (string=w609:string)
                n145 = String To IP(1:w604) -> (0:w603:u32)
                n146 = Concatenate Strings("#C", w609) -> (w606:string)
                n147 = UDP Write(address=w603, port or service name=w605, connection ID=w600, data in=w606, 8:w597, 9:250 ("timeout ms (25000)")) -> (error out=w602:errorcluster, 3:w599:refnum<k16>)
                n148 = call "Wakeup Helper Loop.vi"("Acquisition Types.Acq Types"=T32."CNV Demo", "error in (no error)"=w602, "WiBCI16T Data out"=w586, "connection UDP"=w599, "En MAP"=w587) -> ("error out"=w598:errorcluster)  [unwired: 6 in]
              }
              frame True {
                n149 = call <vilib>:"Clear Errors.vi"("error in (no error)"=w611) -> ("error out"=w610:errorcluster)  [unwired: 5 in, 1 out]
              }
            }
            n150 = Bundle By Name(cluster=w580, "connection UDP"=w581) -> (w579:T1)
          }
          frame "Start EOC Acquiring" {
            # "Acquire EOC Live Data"
            n151 = Variant To Data(error in=w625, type=T28 {"Boolean"=FALSE} ("Start EOC Acquiring Argument"), Variant=w624) -> (error out=w618:errorcluster)  [unwired: 1 out]
            n152 = call "Update Application Settings.vi"("error in"=w618) -> ("error out"=w617:errorcluster, "timed out?"=w616:bool, "Reply Payload"=w615:T14)  [unwired: 8 in]
            n153 = Unbundle By Name(w621) -> ("connection UDP"=w623:refnum<k16>, "WiBCI16T Data"=w614:T4)
            n154 = case shown="True" w616 {
              tunnel: w623 -> [w641 w653]
              tunnel: [w640 w653] -> w622
              tunnel: [w639 w651] -> w619
              tunnel: w617 -> [w638 w652]
              tunnel: w615 -> [w637 _]
              tunnel: w614 -> [w627 _]
              frame False {
                w645 = "255.255.255.255"  # address
                w646 = u16 61557  # remote port
                n155 = call "Typedef to Ch settings.vi"("Reply Payload"=w637) -> ("Referenced Channels"=w635:u16, "Enabled Channels"=w628:u16)  [unwired: 9 in]
                n156 = Split Number(x=w628) -> (hi(x)=w630:u8, lo(x)=w631:u8)
                n157 = Split Number(x=w635) -> (hi(x)=w634:u8, lo(x)=w633:u8)
                n158 = Build Array(w630, w631) -> (w629:u8[])
                n159 = Build Array(w634, w633) -> (w632:u8[])
                n160 = Build Array (concatenate)(u8[] [3] ("unsigned byte array"), w632, w629) -> (w636:u8[])
                n161 = Byte Array To String(unsigned byte array=w636) -> (string=w650:string)
                n162 = String To IP(1:w645) -> (0:w644:u32)
                n163 = Concatenate Strings("#C", w650) -> (w647:string)
                n164 = UDP Write(address=w644, port or service name=w646, connection ID=w641, data in=w647, 8:w638, 9:250 ("timeout ms (25000)")) -> (error out=w643:errorcluster, 3:w640:refnum<k16>)
                n165 = call "Wakeup Helper Loop.vi"("Acquisition Types.Acq Types"=T32."Eyes O/C", "error in (no error)"=w643, "WiBCI16T Data out"=w627, "connection UDP"=w640, "En MAP"=w628) -> ("error out"=w639:errorcluster)  [unwired: 6 in]
              }
              frame True {
                n166 = call <vilib>:"Clear Errors.vi"("error in (no error)"=w652) -> ("error out"=w651:errorcluster)  [unwired: 5 in, 1 out]
              }
            }
            n167 = Bundle By Name(cluster=w621, "connection UDP"=w622) -> (w620:T1)
          }
          frame "Command_ImpedanceData" {
            # "Send Command for Impedance Data with Settings saved"
            n168 = Variant To Data(error in=w666, type=T21 {"Boolean"=FALSE} ("Command_ImpedanceData Argument"), Variant=w665) -> (error out=w655:errorcluster)  [unwired: 1 out]
            n169 = call "Update Application Settings.vi"("error in"=w655) -> ("error out"=w661:errorcluster, "timed out?"=w660:bool, "Reply Payload"=w659:T14)  [unwired: 8 in]
            n170 = Unbundle By Name(w658) -> ("connection UDP"=w663:refnum<k16>, "WiBCI16T Data"=w654:T4)
            n171 = case shown="False" w660 {
              tunnel: w663 -> [w683 w694]
              tunnel: [w682 w694] -> w662
              tunnel: [w667 w693] -> w656
              tunnel: w661 -> [w681 w693]
              tunnel: w659 -> [w680 _]
              tunnel: w654 -> [w670 _]
              frame False {
                w687 = "255.255.255.255"  # address
                w688 = u16 61557  # remote port
                n172 = call "Typedef to Ch settings.vi"("Reply Payload"=w680) -> ("Referenced Channels"=w678:u16, "Enabled Channels"=w671:u16)  [unwired: 9 in]
                n173 = Split Number(x=w671) -> (hi(x)=w673:u8, lo(x)=w674:u8)
                n174 = Split Number(x=w678) -> (hi(x)=w677:u8, lo(x)=w676:u8)
                n175 = Build Array(w673, w674) -> (w672:u8[])
                n176 = Build Array(w677, w676) -> (w675:u8[])
                n177 = Build Array (concatenate)(u8[] [6] ("unsigned byte array"), w675, w672) -> (w679:u8[])
                n178 = Byte Array To String(unsigned byte array=w679) -> (string=w692:string)
                n179 = String To IP(1:w687) -> (0:w686:u32)
                n180 = Concatenate Strings("#C", w692) -> (w689:string)
                n181 = UDP Write(address=w686, port or service name=w688, connection ID=w683, data in=w689, 8:w681, 9:250 ("timeout ms (25000)")) -> (error out=w685:errorcluster, 3:w682:refnum<k16>)
                n182 = call "Wakeup Helper Loop.vi"("Acquisition Types.Acq Types"=T32."Graph", "error in (no error)"=w685, "WiBCI16T Data out"=w670, "connection UDP"=w682, "En MAP"=w671) -> ("error out"=w668:errorcluster)  [unwired: 6 in]
                n183 = call "Wake-up Helper Loop for Pkt Loss Calc.vi"("error in"=w668) -> ("error out"=w667:errorcluster)  [unwired: 10 in]
              }
              frame True {
              }
            }
            n184 = Bundle By Name(cluster=w658, "connection UDP"=w662) -> (w657:T1)
          }
          frame "Start IMP Acquiring" {
            # "Send Command for Impedance Data with Settings saved"
            n185 = Variant To Data(error in=w707, type=T24 {"Boolean"=FALSE} ("Start IMP Acquiring Argument"), Variant=w706) -> (error out=w697:errorcluster)  [unwired: 1 out]
            n186 = call "Update Application Settings.vi"("error in"=w697) -> ("error out"=w703:errorcluster, "timed out?"=w702:bool, "Reply Payload"=w701:T14)  [unwired: 8 in]
            n187 = Unbundle By Name(w700) -> ("connection UDP"=w705:refnum<k16>, "WiBCI16T Data"=w696:T4)
            n188 = case shown="False" w702 {
              tunnel: w705 -> [w723 w735]
              tunnel: [w722 w735] -> w704
              tunnel: [w721 w733] -> w698
              tunnel: w703 -> [w720 w734]
              tunnel: w701 -> [w719 _]
              tunnel: w696 -> [w709 _]
              frame False {
                w727 = "255.255.255.255"  # address
                w728 = u16 61557  # remote port
                n189 = call "Typedef to Ch settings.vi"("Reply Payload"=w719) -> ("Referenced Channels"=w717:u16, "Enabled Channels"=w710:u16)  [unwired: 9 in]
                n190 = Split Number(x=w710) -> (hi(x)=w712:u8, lo(x)=w713:u8)
                n191 = Split Number(x=w717) -> (hi(x)=w716:u8, lo(x)=w715:u8)
                n192 = Build Array(w712, w713) -> (w711:u8[])
                n193 = Build Array(w716, w715) -> (w714:u8[])
                n194 = Build Array (concatenate)(u8[] [6] ("unsigned byte array"), w714, w711) -> (w718:u8[])
                n195 = Byte Array To String(unsigned byte array=w718) -> (string=w732:string)
                n196 = String To IP(1:w727) -> (0:w726:u32)
                n197 = Concatenate Strings("#C", w732) -> (w729:string)
                n198 = UDP Write(address=w726, port or service name=w728, connection ID=w723, data in=w729, 8:w720, 9:250 ("timeout ms (25000)")) -> (error out=w725:errorcluster, 3:w722:refnum<k16>)
                n199 = call "Wakeup Helper Loop.vi"("Acquisition Types.Acq Types"=T32."Impedance", "error in (no error)"=w725, "WiBCI16T Data out"=w709, "connection UDP"=w722, "En MAP"=w710) -> ("error out"=w721:errorcluster)  [unwired: 6 in]
              }
              frame True {
                n200 = call <vilib>:"Clear Errors.vi"("error in (no error)"=w734) -> ("error out"=w733:errorcluster)  [unwired: 5 in, 1 out]
              }
            }
            n201 = Bundle By Name(cluster=w700, "connection UDP"=w704) -> (w699:T1)
          }
          frame "Start GND Loop acquiring" {
            # "Send Command for Impedance Data with Settings saved"
            n202 = Variant To Data(error in=w748, type=T26 {"Boolean"=FALSE} ("Start GND Loop acquiring Argument"), Variant=w747) -> (error out=w738:errorcluster)  [unwired: 1 out]
            n203 = call "Update Application Settings.vi"("error in"=w738) -> ("error out"=w744:errorcluster, "timed out?"=w743:bool, "Reply Payload"=w742:T14)  [unwired: 8 in]
            n204 = Unbundle By Name(w741) -> ("connection UDP"=w746:refnum<k16>, "WiBCI16T Data"=w737:T4)
            n205 = case shown="True" w743 {
              tunnel: w746 -> [w764 w776]
              tunnel: [w763 w776] -> w745
              tunnel: [w762 w774] -> w739
              tunnel: w744 -> [w761 w775]
              tunnel: w742 -> [w760 _]
              tunnel: w737 -> [w750 _]
              frame False {
                w768 = "255.255.255.255"  # address
                w769 = u16 61557  # remote port
                n206 = call "Typedef to Ch settings.vi"("Reply Payload"=w760) -> ("Referenced Channels"=w758:u16, "Enabled Channels"=w751:u16)  [unwired: 9 in]
                n207 = Split Number(x=w751) -> (hi(x)=w753:u8, lo(x)=w754:u8)
                n208 = Split Number(x=w758) -> (hi(x)=w757:u8, lo(x)=w756:u8)
                n209 = Build Array(w753, w754) -> (w752:u8[])
                n210 = Build Array(w757, w756) -> (w755:u8[])
                n211 = Build Array (concatenate)(u8[] [8] ("unsigned byte array"), w755, w752) -> (w759:u8[])
                n212 = Byte Array To String(unsigned byte array=w759) -> (string=w773:string)
                n213 = String To IP(1:w768) -> (0:w767:u32)
                n214 = Concatenate Strings("#C", w773) -> (w770:string)
                n215 = UDP Write(address=w767, port or service name=w769, connection ID=w764, data in=w770, 8:w761, 9:250 ("timeout ms (25000)")) -> (error out=w766:errorcluster, 3:w763:refnum<k16>)
                n216 = call "Wakeup Helper Loop.vi"("Acquisition Types.Acq Types"=T32."Impedance", "error in (no error)"=w766, "WiBCI16T Data out"=w750, "connection UDP"=w763, "En MAP"=w751) -> ("error out"=w762:errorcluster)  [unwired: 6 in]
              }
              frame True {
                n217 = call <vilib>:"Clear Errors.vi"("error in (no error)"=w775) -> ("error out"=w774:errorcluster)  [unwired: 5 in, 1 out]
              }
            }
            n218 = Bundle By Name(cluster=w741, "connection UDP"=w745) -> (w740:T1)
          }
          frame "Command_GoToIdle" {
            w788 = "255.255.255.255"  # address
            w789 = u16 61557  # remote port
            # "Go toIDLE command as per API 2.5"
            n219 = Variant To Data(error in=w796, type=T22 {"Boolean"=FALSE} ("Command_GoToIdle Argument"), Variant=w795) -> (error out=w783:errorcluster)  [unwired: 1 out]
            n220 = Unbundle By Name(w780) -> ("connection UDP"=w786:refnum<k16>)
            n221 = Byte Array To String(unsigned byte array=u8[] [1, 0, 0, 0, 0]) -> (string=w793:string)
            n222 = String To IP(1:w788) -> (0:w787:u32)
            n223 = Concatenate Strings("#C", w793) -> (w790:string)
            n224 = UDP Write(address=w787, port or service name=w789, connection ID=w786, data in=w790, 8:w783, 9:250 ("timeout ms (25000)")) -> (error out=w782:errorcluster, 3:w785:refnum<k16>)
            n225 = call-poly <userlib>:"MGI Wait.vi"("ms"=u32 5, "Error In"=w782) -> ("Error Out"=w777:errorcluster)  [unwired: 5 in]
            n226 = Bundle By Name(cluster=w780, "connection UDP"=w785) -> (w781:T1)
            n227 = call "Status Updated.vi"("error in (no error)"=w777, "Status"="Acquisition Stopped") -> ()  [unwired: 9 in, 1 out]
            n228 = call "Acquisition Stopped.vi"("error in (no error)"=w777) -> ()  [unwired: 10 in, 1 out]
            n229 = call "Stop Pkt Loss Calc.vi"("error in"=w777) -> ()  [unwired: 10 in, 1 out]
          }
          frame "Soft Trigger" {
            # "UI is sending Soft Trigger to Acquisition Module"
            n230 = Variant To Data(error in=w802, type=T23 {"Value"=0} ("Soft Trigger Argument"), Variant=w800) -> (error out=w798:errorcluster)  [unwired: 1 out]
            n231 = call "Status Updated.vi"("error in (no error)"=w798, "Status"="Soft Trigger Initiated ...") -> ()  [unwired: 9 in, 1 out]
          }
          frame "Stop IMP acquiring" {
            # "Stops acquiring Impedance Data"
            n232 = Variant To Data(error in=w807, type=T25 {"Boolean"=FALSE} ("Stop IMP acquiring Argument"), Variant=w804) -> (error out=w805:errorcluster)  [unwired: 1 out]
          }
          frame "Command_GndImpedanceData" {
            # "#CodeNeeded\n1. Configure this Message Case for handling the \"Command_GndImpedanceData\" message.\n2. Delete or edit this label when done."
            # "Command for gnd impedance mode"
            n233 = Variant To Data(error in=w813, type=T29 {"Boolean"=FALSE} ("Command_GndImpedanceData Argument"), Variant=w810) -> (data=w808:T29, error out=w811:errorcluster)
            n234 = Unbundle By Name(w808) -> ()  [unwired: 1 out]
          }
          frame "---Copy This Frame---" {
            # "Duplicate this frame when creating new messages.  Change this comment in the duplicated frame to describe this message."
            n235 = Merge Errors(w816) -> (w815:errorcluster)
          }
          frame "Check WiFi AP" {
            w820 = u16 61557  # remote port
            w832 = "255.255.255.255"  # address
            w842 = u16 61556  # local port
            # "Max of 5 Attempts ..."
            # "Check WiFi connection with WiBCI amplifier. If connected, Proceed.\nIf not, Show User warning and Exit ..."
            n236 = Variant To Data(error in=w823, type=T18 {"Connected ?"=FALSE} ("Check WiFi AP Argument"), Variant=w824) -> ()  [unwired: 2 out]
            n237 = Byte Array To String(unsigned byte array=u8[] [241, 0, 0, 0, 0]) -> (string=w835:string)
            n238 = UDP Open(8:w823, 9:100 ("timeout ms (25000)"), 11:w842) -> (port=w822:refnum<k16>, 0:w839:errorcluster)  [unwired: 2 in, 1 out]
            n239 = Concatenate Strings("#C", w835) -> (w834:string)
            n240 = String To IP(1:w832) -> (0:w819:u32)
            n241 = call-poly <userlib>:"MGI Wait.vi"("ms"=u32 10, "Error In"=w839) -> ("Error Out"=w833:errorcluster)  [unwired: 5 in]
            n242 = for {
              N: 5 -> [_]
              tunnel: 250 ("timeout ms (25000)") -> [w874]
              tunnel: w834 -> [w873]
              tunnel: w822 -> [w872]
              tunnel: w833 -> [w871]
              tunnel: w819 -> [w870]
              tunnel: w820 -> [w869]
              tunnel: [w861] -> w830
              tunnel: [w860] -> w821
              tunnel: [w859] -> w818
              tunnel: [w858] -> w817
              n243 = UDP Write(address=w870, port or service name=w869, connection ID=w872, data in=w873, 8:w871, 9:w874) -> (error out=w866:errorcluster, 3:w867:refnum<k16>)
              n244 = Wait Until Next ms Multiple(millisecond multiple=u32 150) -> ()  [unwired: 1 out]
              n245 = UDP Read(connection ID=w867, timeout ms (25000)=100, 8:w866) -> (data out=w858:string, error out=w860:errorcluster, 3:w859:refnum<k16>)  [unwired: 3 out]
              n246 = String Subset(string=w858, length (rest)=2 ("length (rest)")) -> (substring=w864:string)  [unwired: 1 in]
              n247 = Equal?(x="$S", y=w864) -> (x = y?=w861:bool)
            }
            n248 = call <vilib>:"Clear Errors.vi"("error in (no error)"=w821) -> ("error out"=w826:errorcluster)  [unwired: 5 in, 1 out]
            n249 = case shown="True" w830 {
              tunnel: w829 -> [w846 w855]
              tunnel: w826 -> [w845 w852]
              tunnel: [w846 w857] -> w828
              tunnel: w818 -> [_ w856]
              tunnel: [w844 w851] -> w827
              tunnel: w817 -> [_ w853]
              frame False {
                n250 = call "STOP_GUI.vi"("error in"=w845, "Message for the Request"="System is not connected to WiBCI Wi-Fi Access Point") -> ("error out"=w844:errorcluster)  [unwired: 9 in]
              }
              frame True {
                n251 = Unbundle By Name(w855) -> ("WiBCI16T Data"=w854:T4)
                n252 = call "Decode and Update.vi"("error in"=w852, "WiBCI16T Data"=w854, "data in"=w853, "Data Valid ?"=TRUE) -> ("error out"=w851:errorcluster, "WiBCI16T Data out"=w847:T4)  [unwired: 6 in]
                n253 = Bundle By Name(cluster=w855, "connection UDP"=w856, "WiBCI16T Data"=w847) -> (w857:T1)
                n254 = call "Data Updated.vi"("En MAP"=u16 0, "WiBCI16T Data in"=w847) -> ("error out"=w848:errorcluster)  [unwired: 9 in]
                n255 = call <vilib>:"Clear Errors.vi"("error in (no error)"=w848) -> ()  [unwired: 5 in, 2 out]
              }
            }
          }
          frame "---Exit and Error Handling---" {
            # "Separator - The following cases handle errors and exit messages."
          }
          frame "Error" {
            # "Error - Check the error message data and respond accordingly. This message is sent by the \"Error Handler\" VIs at the end of each loop in this application."
            n256 = property class="Module Admin"(reference=w878) -> ("Accessors:External Launch"=w877:bool)  [unwired: 1 in, 2 out]
            n257 = Variant To Data(error in=w886, type=errorcluster {"status"=FALSE, "code"=0, "source"=""} ("error constant"), Variant=w880) -> (data=w887:errorcluster, error out=w884:errorcluster)
            n258 = call "Error Reported.vi"("Error"=w887) -> ()  [unwired: 10 in, 1 out]
            n259 = case shown="False" w877 {
              tunnel: [w892 _] -> w883
              tunnel: w879 -> [w890 _]
              tunnel: w887 -> [w891 _]
              frame False {
                # "If the module is running standalone, then pop up an error dialog and call the \"Exit\" message."
                n260 = call <vilib>:"Simple Error Handler.vi"("error in (no error)"=w891) -> ()  [unwired: 4 in, 5 out]
                n261 = call-poly <vilib>:"Delacor_lib_QMH_Enqueue Message (poly).vi"("Priority Message? (F)"=TRUE, "Message"="Exit", "Message Queue in"=w890) -> ("error out"=w892:errorcluster)  [unwired: 7 in, 1 out]
              }
              frame True {
                # "If the module was launched externally, calling the Error Reported broadcast VI is the only action performed by the \"Error\" message. The module's caller can then process the error appropriately."
              }
            }
            n262 = Merge Errors(w884, w883) -> (w882:errorcluster)
            n263 = local write "error out"(w882) -> ()
          }
          frame "Exit" {
            w900 = 91  # 91: not all Exit messages will have an argument
            w902 = TRUE  # Stop the VI
            # "Release the message queue reference"
            # "Exit - Exit the application."
            n264 = Variant To Data(error in=w910, type=T11 {"Origin"="", "Exit via Stop Module Req?"=FALSE, "Wait for Module to stop?"=FALSE} ("Stop Argument"), Variant=w901) -> (data=w898:T11, error out=w906:errorcluster)
            n265 = call <vilib>:"Clear Errors.vi"("error in (no error)"=w906, "specific error code to clear (0: all)"=w900) -> ("error out"=w909:errorcluster)  [unwired: 4 in, 1 out]
            n266 = Unbundle By Name(w895) -> ("connection UDP"=w893:refnum<k16>)
            n267 = control-ref of="This VI"() -> (w897:refnum<vi>)
            n268 = call "Handle Exit.vi"("Stop Argument"=w898, "Admin in"=w896, "VI reference"=w897) -> ("error out"=w905:errorcluster)  [unwired: 7 in, 1 out]
            n269 = call-dynamic "Delacor_lib_QMH_Release Message Queue.vi"("error in"=w909, "Message Queue"=w903) -> ("error out"=w908:errorcluster)  [unwired: 9 in]
            n270 = call "Close Hardware References.vi"("connection ID in"=w893) -> ("error out"=w904:errorcluster)  [unwired: 9 in, 1 out]
            n271 = Merge Errors(w908, w905, w904) -> (w907:errorcluster)
            n272 = case "Settings Editor was\nalready running?" shown="False" w894 {
              frame False {
                n273 = call "Module Name--constant.vi"() -> ("Module Name"=w912:string)  [unwired: 11 in]
                n274 = call "Stop Module.vi"("Wait for Module to Stop? (F)"=TRUE, "Origin"=w912) -> ()  [unwired: 9 in, 1 out]
              }
              frame True {
                # "Another Module is\nin charge of stopping Settings Editor"
              }
            }
            n275 = call "Error Reported.vi"("Error"=w907) -> ()  [unwired: 10 in, 1 out]
          }
          frame Default {
            # "'Default' case only runs if there is a message that isn't defined in any of the other cases.  Output a programming error."
            n276 = call "Module Name--constant.vi"() -> ("Module Name"=w913:string)  [unwired: 11 in]
            n277 = xnode "Error Ring"("parameter 0"=w914, "parameter 1"=w913) -> ("error out"=w916:errorcluster)
            n278 = Merge Errors(w917, w916) -> (w918:errorcluster)
          }
        }
        "Settings" <- w407
        n279 = call-dynamic "Delacor_lib_QMH_Error Handler - Message Handling Loop.vi"("error in"=w412, "Message Queue in"=w402) -> ("dup error in"=w409:errorcluster)  [unwired: 8 in, 1 out]
      }
      n280 = while {
        tunnel: w41 -> [w258]
        shift-right: [w261] -> w46
        shift-left: w45 -> [w262]
        tunnel: [w263] -> w48
        tunnel: w44 -> [w259]
        stop <- w260 stop-if-true
        # "Event Handling Loop"
        n281 = event "DQMH_EVENT_MAIN" shown="[21] <Acquisition Request Events.Command_GndImpedanceData>: User Event" {
          selector: w262 -> [_ _ _ _ _ _ _ _ _ _ _ _ _ _ _ _ _ _ _ _ _ _]
          dyn-events: [_ _ _ _ _ _ _ _ _ _ _ _ _ _ _ _ _ _ _ _ _ _] -> w261
          timeout: _ -> [_ _ _ _ _ _ _ _ _ _ _ _ _ _ _ _ _ _ _ _ _ _]
          tunnel: [_ _ _ _ TRUE ("Discard?") _ _ _ _ _ _ _ _ _ _ _ _ _ _ _ _ _] -> w260
          tunnel: w258 -> [_ _ _ _ w286 w293 w309 w314 w319 w327 w333 w339 w345 w351 w357 w363 w369 w375 w381 w387 w393 w399]
          tunnel: [_ _ w270 _ w289 w295 w305 w315 w321 w322 w328 w334 w340 w346 w352 w358 w364 w370 w376 w382 w388 w394] -> w264
          tunnel: w259 -> [_ _ _ _ _ w292 _ _ _ _ _ _ _ _ _ _ _ _ _ _ _ _]
          event User Event {
            # "Show the panel of this VI, and send a status updated message to let listeners know."
            # "Another Module called the \"Show Panel\" API Method."
            n282 = event-data() -> ()  [unwired: 1 in, 1 out]
            n283 = control-ref of="This VI"() -> (w266:refnum<vi>)
            n284 = call "Open VI Panel.vi"("VI"=w266) -> ()  [unwired: 10 in, 1 out]
            n285 = call "Status Updated.vi"("Status"="Panel shown." ("format string")) -> ()  [unwired: 10 in, 1 out]
          }
          event User Event {
            # "Hide the panel of this VI, and send a status updated message to let listeners know."
            # "Another Module called the \"Hide Panel\" API Method."
            n286 = event-data() -> ()  [unwired: 1 in, 1 out]
            n287 = control-ref of="This VI"() -> (w268:refnum<vi>)
            n288 = call "Hide VI Panel.vi"("VI"=w268) -> ()  [unwired: 10 in, 1 out]
            n289 = call "Status Updated.vi"("Status"="Panel hidden." ("format string")) -> ()  [unwired: 10 in, 1 out]
          }
          event User Event {
            # "Another Module called the \"Get Module Execution Status\" API Method."
            n290 = event-data() -> ()  [unwired: 1 in, 1 out]
            n291 = call "Update Module Execution Status.vi"("Running?"=TRUE) -> ("error out"=w270:errorcluster)  [unwired: 10 in]
          }
          event User Event {
            # "Another Module called the \"Show Diagram\" API Method. This event is used for debugging."
            n292 = event-data() -> ()  [unwired: 1 in, 1 out]
            n293 = disable-structure shown="RUN_TIME_ENGINE==False" {
              frame condition #0 (active) {
                # "functionality not available in exe"
                n294 = invoke class="VI" method="Lock State.Get"() -> (error out=w276:errorcluster, "Get Lock State"=w275:T10, "pwd in cache"=w272:bool)  [unwired: 4 in, 1 out]
                n295 = Equal?(x=T10."Password-protected", y=w275) -> (x = y?=w273:bool)
                n296 = Compound Arithmetic op=AND(w273, invert w272) -> (w271:bool)
                n297 = case shown="False" w271 {
                  tunnel: w276 -> [w279 _]
                  frame False {
                    n298 = property class="VI"(error in=w279, "BDWin.Open"=TRUE ("Block Diagram Window:Open")) -> ()  [unwired: 1 in, 2 out]
                    n299 = call "Status Updated.vi"("Status"="Block Diagram shown." ("format string")) -> ()  [unwired: 10 in, 1 out]
                  }
                  frame True {
                    # "Password-protected VI, and the password is not in the cache. Do not show the diagram."
                  }
                }
              }
              frame condition #1 {
              }
            }
          }
          event User Event {
            # "The Stop Module Event can get fired from the Exit message in the MHL. The queue gets destroyed in that case. If the queue no longer exists, the Enqueue Exit as a priority message will return error 1. Ignoring because the module is already exiting."
            # "Another Module called the \"Stop Module\" API Method  or the Message Handling Loop below."
            n300 = event-data() -> ("Exit via Stop Module Req?"=w282:bool, "Wait for Module to stop?"=w281:bool)  [unwired: 1 in]
            n301 = Bundle By Name(cluster=T11 {"Origin"="", "Exit via Stop Module Req?"=FALSE, "Wait for Module to stop?"=FALSE} ("Stop Argument"), "Exit via Stop Module Req?"=w282, "Wait for Module to stop?"=w281) -> (w280:T11)
            n302 = call-poly <vilib>:"Delacor_lib_QMH_Enqueue Message (poly).vi"("Priority Message? (F)"=TRUE, "Message Data"=w280, "Message"="Exit", "Message Queue in"=w286) -> ("error out"=w290:errorcluster)  [unwired: 6 in, 1 out]
            n303 = call <vilib>:"Clear Errors.vi"("error in (no error)"=w290, "specific error code to clear (0: all)"=1) -> ("error out"=w289:errorcluster)  [unwired: 4 in, 1 out]
          }
          event Panel Close? {
            w294 = TRUE  # Discard the event, the MHL is responsible for closing and stopping this VI.
            # "Hide the panel or send the 'Exit' message if the user clicks the 'X' on the module main VI panel."
            n304 = event-data() -> ()  [unwired: 1 in, 1 out]
            n305 = property class="Module Admin"(reference=w292) -> ("Accessors:External Launch"=w291:bool)  [unwired: 1 in, 2 out]
            n306 = case shown="False" w291 {
              tunnel: w293 -> [_ w301]
              tunnel: [_ w302] -> w295
              frame True {
                # "If externally launched, clicking the 'X' hides the panel, but doesn't close it."
                n307 = control-ref of="This VI"() -> (w298:refnum<vi>)
                n308 = call "Hide VI Panel.vi"("VI"=w298) -> ("error out"=w296:errorcluster)  [unwired: 10 in]
                n309 = call "Status Updated.vi"("error in (no error)"=w296, "Status"="Panel hidden.") -> ()  [unwired: 9 in, 1 out]
              }
              frame False {
                # "If run as a stand-alone VI, clicking the panel 'X' stops the VI."
                n310 = call-poly <vilib>:"Delacor_lib_QMH_Enqueue Message (poly).vi"("Priority Message? (F)"=TRUE, "Message"="Exit", "Message Queue in"=w301) -> ("error out"=w302:errorcluster)  [unwired: 7 in, 1 out]
              }
            }
            n311 = event-data("Discard?"=w294) -> ()  [unwired: 1 in, 1 out]
          }
          event User Event {
            # "Another Module called the \"Start Acquiring\" API Method."
            n312 = event-data() -> ("Wait Notifier"=w304:refnum<notifier>, "wait for reply"=w303:bool)  [unwired: 1 in]
            n313 = Bundle(cluster=T12 {"Wait Notifier"=refnum, "wait for reply"=FALSE} ("Start Acquisition Argument"), "Wait Notifier"=w304, "wait for reply"=w303) -> (w306:T12)
            n314 = call-poly <vilib>:"Delacor_lib_QMH_Enqueue Message (poly).vi"("Message Data"=w306, "Message"="Start Acquiring", "Message Queue in"=w309) -> ("error out"=w305:errorcluster)  [unwired: 7 in, 1 out]
          }
          event User Event {
            # "Another Module called the \"Stop Acquiring\" API Method."
            n315 = event-data() -> ("Boolean"=w310:bool)  [unwired: 1 in]
            n316 = Bundle(cluster=T13 {"Boolean"=FALSE} ("Stop Acquiring Argument"), "Boolean"=w310) -> (w311:T13)
            n317 = call-poly <vilib>:"Delacor_lib_QMH_Enqueue Message (poly).vi"("Message Data"=w311, "Message"="Stop Acquiring", "Message Queue in"=w314) -> ("error out"=w315:errorcluster)  [unwired: 7 in, 1 out]
          }
          event User Event {
            n318 = event-data() -> ("Settings"=w316:T15)  [unwired: 1 in]
            n319 = Bundle By Name(cluster=T14 {"Settings"={"Signal Type"=enum."Sine Wave", "Calibration Array"=[], "Log File Base Path"=path "", "EEG Channels"={"16 EEG Channels"=[], "Gain"=24}, "Soft Trig enum"=enum."Disable Soft Trigger", "Montage selection"={"Montages Ref"=refnum, "Selected Montage Number"=0, "Montages Names"=[]}, "LSL En enum"=enum."LSL Disabled"}, "error"={"status"=FALSE, "code"=0, "source"=""}} ("Settings Updated Argument"), "Settings"=w316) -> (w318:T14)
            n320 = call-poly <vilib>:"Delacor_lib_QMH_Enqueue Message (poly).vi"("Message Data"=w318, "Message"="Update Settings", "Message Queue in"=w319) -> ("error out"=w321:errorcluster)  [unwired: 7 in, 1 out]
          }
          event User Event {
            # "Another Module called the \"Command_TestData\" API Method."
            n321 = event-data() -> ("Boolean"=w323:bool)  [unwired: 1 in]
            n322 = Bundle(cluster=T17 {"Boolean"=FALSE} ("Command_TestData Argument"), "Boolean"=w323) -> (w324:T17)
            n323 = call-poly <vilib>:"Delacor_lib_QMH_Enqueue Message (poly).vi"("Message Data"=w324, "Message"="Command_TestData", "Message Queue in"=w327) -> ("error out"=w322:errorcluster)  [unwired: 7 in, 1 out]
          }
          event User Event {
            # "Another Module called the \"Check WiFi AP\" API Method."
            n324 = event-data() -> ("Connected ?"=w329:bool)  [unwired: 1 in]
            n325 = Bundle(cluster=T18 {"Connected ?"=FALSE} ("Check WiFi AP Argument"), "Connected ?"=w329) -> (w330:T18)
            n326 = call-poly <vilib>:"Delacor_lib_QMH_Enqueue Message (poly).vi"("Message Data"=w330, "Message"="Check WiFi AP", "Message Queue in"=w333) -> ("error out"=w328:errorcluster)  [unwired: 7 in, 1 out]
          }
          event User Event {
            # "Another Module called the \"Command_NoiseData\" API Method."
            n327 = event-data() -> ("Boolean"=w335:bool)  [unwired: 1 in]
            n328 = Bundle(cluster=T19 {"Boolean"=FALSE} ("Command_NoiseData Argument"), "Boolean"=w335) -> (w336:T19)
            n329 = call-poly <vilib>:"Delacor_lib_QMH_Enqueue Message (poly).vi"("Message Data"=w336, "Message"="Command_NoiseData", "Message Queue in"=w339) -> ("error out"=w334:errorcluster)  [unwired: 7 in, 1 out]
          }
          event User Event {
            # "Another Module called the \"Command_LiveData\" API Method."
            n330 = event-data() -> ("Boolean"=w341:bool)  [unwired: 1 in]
            n331 = Bundle(cluster=T20 {"Boolean"=FALSE} ("Command_LiveData Argument"), "Boolean"=w341) -> (w342:T20)
            n332 = call-poly <vilib>:"Delacor_lib_QMH_Enqueue Message (poly).vi"("Message Data"=w342, "Message"="Command_LiveData", "Message Queue in"=w345) -> ("error out"=w340:errorcluster)  [unwired: 7 in, 1 out]
          }
          event User Event {
            # "Another Module called the \"Command_ImpedanceData\" API Method."
            n333 = event-data() -> ("Boolean"=w347:bool)  [unwired: 1 in]
            n334 = Bundle(cluster=T21 {"Boolean"=FALSE} ("Command_ImpedanceData Argument"), "Boolean"=w347) -> (w348:T21)
            n335 = call-poly <vilib>:"Delacor_lib_QMH_Enqueue Message (poly).vi"("Message Data"=w348, "Message"="Command_ImpedanceData", "Message Queue in"=w351) -> ("error out"=w346:errorcluster)  [unwired: 7 in, 1 out]
          }
          event User Event {
            # "Another Module called the \"Command_GoToIdle\" API Method."
            n336 = event-data() -> ("Boolean"=w353:bool)  [unwired: 1 in]
            n337 = Bundle(cluster=T22 {"Boolean"=FALSE} ("Command_GoToIdle Argument"), "Boolean"=w353) -> (w354:T22)
            n338 = call-poly <vilib>:"Delacor_lib_QMH_Enqueue Message (poly).vi"("Message Data"=w354, "Message"="Command_GoToIdle", "Message Queue in"=w357) -> ("error out"=w352:errorcluster)  [unwired: 7 in, 1 out]
          }
          event User Event {
            # "Another Module called the \"Soft Trigger\" API Method."
            n339 = event-data() -> ("Value"=w359:i8)  [unwired: 1 in]
            n340 = Bundle(cluster=T23 {"Value"=0} ("Soft Trigger Argument"), "Value"=w359) -> (w360:T23)
            n341 = call-poly <vilib>:"Delacor_lib_QMH_Enqueue Message (poly).vi"("Message Data"=w360, "Message"="Soft Trigger", "Message Queue in"=w363) -> ("error out"=w358:errorcluster)  [unwired: 7 in, 1 out]
          }
          event User Event {
            # "Another Module called the \"Start IMP Acquiring\" API Method."
            n342 = event-data() -> ("Boolean"=w365:bool)  [unwired: 1 in]
            n343 = Bundle(cluster=T24 {"Boolean"=FALSE} ("Start IMP Acquiring Argument"), "Boolean"=w365) -> (w366:T24)
            n344 = call-poly <vilib>:"Delacor_lib_QMH_Enqueue Message (poly).vi"("Message Data"=w366, "Message"="Start IMP Acquiring", "Message Queue in"=w369) -> ("error out"=w364:errorcluster)  [unwired: 7 in, 1 out]
          }
          event User Event {
            # "Another Module called the \"Stop IMP acquiring\" API Method."
            n345 = event-data() -> ("Boolean"=w371:bool)  [unwired: 1 in]
            n346 = Bundle(cluster=T25 {"Boolean"=FALSE} ("Stop IMP acquiring Argument"), "Boolean"=w371) -> (w372:T25)
            n347 = call-poly <vilib>:"Delacor_lib_QMH_Enqueue Message (poly).vi"("Message Data"=w372, "Message"="Stop IMP acquiring", "Message Queue in"=w375) -> ("error out"=w370:errorcluster)  [unwired: 7 in, 1 out]
          }
          event User Event {
            # "Another Module called the \"Start GND Loop acquiring\" API Method."
            n348 = event-data() -> ("Boolean"=w377:bool)  [unwired: 1 in]
            n349 = Bundle(cluster=T26 {"Boolean"=FALSE} ("Start GND Loop acquiring Argument"), "Boolean"=w377) -> (w378:T26)
            n350 = call-poly <vilib>:"Delacor_lib_QMH_Enqueue Message (poly).vi"("Message Data"=w378, "Message"="Start GND Loop acquiring", "Message Queue in"=w381) -> ("error out"=w376:errorcluster)  [unwired: 7 in, 1 out]
          }
          event User Event {
            # "Another Module called the \"Start CNV Acquiring\" API Method."
            n351 = event-data() -> ("Boolean"=w383:bool)  [unwired: 1 in]
            n352 = Bundle(cluster=T27 {"Boolean"=FALSE} ("Start CNV Acquiring Argument"), "Boolean"=w383) -> (w384:T27)
            n353 = call-poly <vilib>:"Delacor_lib_QMH_Enqueue Message (poly).vi"("Message Data"=w384, "Message"="Start CNV Acquiring", "Message Queue in"=w387) -> ("error out"=w382:errorcluster)  [unwired: 7 in, 1 out]
          }
          event User Event {
            # "Another Module called the \"Start EOC Acquiring\" API Method."
            n354 = event-data() -> ("Boolean"=w389:bool)  [unwired: 1 in]
            n355 = Bundle(cluster=T28 {"Boolean"=FALSE} ("Start EOC Acquiring Argument"), "Boolean"=w389) -> (w390:T28)
            n356 = call-poly <vilib>:"Delacor_lib_QMH_Enqueue Message (poly).vi"("Message Data"=w390, "Message"="Start EOC Acquiring", "Message Queue in"=w393) -> ("error out"=w388:errorcluster)  [unwired: 7 in, 1 out]
          }
          event User Event {
            # "Another Module called the \"Command_GndImpedanceData\" API Method."
            n357 = event-data() -> ("Boolean"=w395:bool)  [unwired: 1 in]
            n358 = Bundle(cluster=T29 {"Boolean"=FALSE} ("Command_GndImpedanceData Argument"), "Boolean"=w395) -> (w396:T29)
            n359 = call-poly <vilib>:"Delacor_lib_QMH_Enqueue Message (poly).vi"("Message Data"=w396, "Message"="Command_GndImpedanceData", "Message Queue in"=w399) -> ("error out"=w394:errorcluster)  [unwired: 7 in, 1 out]
          }
        }
        n360 = call-dynamic "Delacor_lib_QMH_Error Handler - Event Handling Loop.vi"("error in"=w264, "Message Queue in"=w258) -> ("dup error in"=w263:errorcluster)  [unwired: 8 in, 1 out]
      }
      n361 = while "DQMH_HELPER_LOOP" {
        shift-right: [w59] -> _
        shift-left: -1 -> [w58]
        shift-right: [w56] -> w36
        shift-left: w35 -> [w57]
        tunnel: w41 -> [w53]
        shift-right: [w50] -> _
        shift-left: w33 -> [w51]
        stop <- w55 stop-if-true
        w52 = "Helper Loop for Pkt Loss Calc"  # DQMH_HELPER_LOOP_NAME
        # "Helper Loop for Pkt Loss Calc"
        n362 = event "DQMH_HELPER_EVENT_STRUCTURE" shown="[5] <Acquisition Request Events.Private.Calculate Packet Loss>: User Event" {
          selector: w57 -> [_ _ _ _ _ _]
          dyn-events: [_ _ _ _ _ _] -> w56
          timeout: w58 -> [_ _ _ _ _ _]
          tunnel: w58 -> [w61 w65 w67 _ w82 w108]
          tunnel: [w61 w65 w67 w75 w82 w108] -> w59
          tunnel: [_ TRUE _ _ _ _] -> w55
          tunnel: [_ errorcluster {"status"=FALSE, "code"=0, "source"=""} ("error constant") _ _ _ _] -> w54
          tunnel: w53 -> [_ _ _ _ _ _]
          tunnel: w51 -> [w60 w62 w71 w73 w81 w105]
          tunnel: [w60 w62 w70 w72 w77 w104] -> w50
          event Timeout {
            n363 = event-data() -> ()  [unwired: 1 in, 1 out]
          }
          event User Event {
            n364 = event-data() -> ()  [unwired: 1 in, 1 out]
          }
          event User Event {
            # "Keep the Helper Loop Sleeping\nNeed to initialise Calc Data"
            # "This module called the \"Private.Wake-up Helper Loop for Pkt Loss Calc\" private request."
            n365 = event-data() -> ()  [unwired: 1 in, 1 out]
            n366 = Bundle By Name(cluster=w71, "Pkt Loss Calc elements.Array"=u32[] [0, 0, 0, 0, 0, 0, 0, 0, 0, 0, 0, 0, 0, 0, 0, 0, 0, 0, 0, 0, 0, 0, 0, 0, 0, 0, 0, 0, 0, 0, 0, 0, 0, 0, 0, 0, 0, 0, 0, 0, 0, 0, 0, 0, 0, 0, 0, 0, 0, 0, 0, 0, 0, 0, 0, 0, 0, 0, 0, 0, 0, 0, 0, 0, 0, 0, 0, 0, 0, 0, 0, 0, 0, 0, 0, 0, 0, 0, 0, 0, 0, 0, 0, 0, 0, 0, 0, 0, 0, 0, 0, 0, 0, 0, 0, 0, 0, 0, 0, 0, 0, 0, 0, 0, 0, 0, 0, 0, 0, 0, 0, 0, 0, 0, 0, 0, 0, 0, 0, 0, 0, 0, 0, 0, 0, 0, 0, 0, 0, 0, 0, 0, 0, 0, 0, 0, 0, 0, 0, 0, 0, 0, 0, 0, 0, 0, 0, 0, 0, 0, 0, 0, 0, 0, 0, 0, 0, 0, 0, 0, 0, 0, 0, 0, 0, 0, 0, 0, 0, 0, 0, 0, 0, 0, 0, 0, 0, 0, 0, 0, 0, 0, 0, 0, 0, 0, 0, 0, 0, 0, 0, 0, 0, 0, 0, 0, 0, 0, 0, 0, 0, 0, 0, 0, 0, 0, 0, 0, 0, 0, 0, 0, 0, 0, 0, 0, 0, 0, 0, 0, 0, 0, 0, 0, 0, 0, 0, 0, 0, 0, 0, 0, 0, 0, 0, 0, 0, 0, 0, 0, 0, 0, 0, 0, 0, 0, 0, 0, 0, 0, 0, 0, 0, 0, 0, 0, 0, 0, 0, 0, 0, 0, 0, 0, 0, 0, 0, 0, 0, 0, 0, 0, 0, 0, 0, 0, 0, 0, 0, 0, 0, 0, 0, 0, 0, 0, 0, 0, 0, 0, 0, 0, 0, 0, 0, 0, 0, 0, 0, 0, 0, 0, 0, 0, 0, 0, 0, 0, 0, 0, 0, 0, 0, 0, 0, 0, 0, 0, 0, 0, 0, 0, 0, 0, 0, 0, 0, 0, 0, 0, 0, 0, 0, 0, 0, 0, 0, 0, 0, 0, 0, 0, 0, 0, 0, 0, 0, 0, 0, 0, 0, 0, 0, 0, 0, 0, 0, 0, 0, 0, 0, 0, 0, 0, 0, 0, 0, 0, 0, 0, 0, 0, 0, 0, 0, 0, 0, 0, 0, 0, 0, 0, 0, 0, 0, 0, 0, 0, 0, 0, 0, 0, 0, 0, 0, 0, 0, 0, 0, 0, 0, 0, 0, 0, 0, 0, 0, 0, 0, 0, 0, 0, 0, 0, 0, 0, 0, 0, 0, 0, 0, 0, 0, 0, 0, 0, 0, 0, 0, 0, 0, 0, 0, 0, 0, 0, 0, 0, 0, 0, 0, 0, 0, 0, 0, 0, 0, 0, 0, 0, 0, 0, 0, 0, 0, 0, 0, 0, 0, 0, 0, 0, 0, 0, 0, 0, 0, 0, 0, 0, 0, 0, 0, 0, 0, 0, 0, 0, 0, 0, 0, 0, 0, 0, 0, 0, 0, 0, 0, 0, 0, 0, 0, 0, 0, 0, 0, 0, 0, 0, 0, 0, 0, 0, 0, 0, 0, 0, 0, 0, 0, 0, 0, 0, 0, 0, 0, 0, 0, 0, 0, 0, 0, 0, 0, 0, 0, 0, 0, 0, 0, 0, 0, 0, 0, 0, 0, 0, 0, 0, 0, 0, 0, 0, 0, 0, 0, 0, 0, 0, 0, 0, 0, 0, 0, 0, 0, 0, 0, 0, 0, 0, 0, 0, 0, 0, 0, 0, 0, 0, 0, 0, 0, 0, 0, 0, 0, 0, 0, 0, 0, 0, 0, 0, 0, 0, 0, 0, 0, 0, 0, 0, 0, 0, 0, 0, 0, 0, 0, 0, 0, 0, 0, 0, 0, 0, 0, 0, 0, 0, 0, 0, 0, 0, 0, 0, 0, 0, 0, 0, 0, 0, 0, 0, 0, 0, 0, 0, 0, 0, 0, 0, 0, 0, 0, 0, 0, 0, 0, 0, 0, 0, 0, 0, 0, 0, 0, 0, 0, 0, 0, 0, 0, 0, 0, 0, 0, 0, 0, 0, 0, 0, 0, 0, 0, 0, 0, 0, 0, 0, 0, 0, 0, 0, 0, 0, 0, 0, 0, 0, 0, 0, 0, 0, 0, 0, 0, 0, 0, 0, 0, 0, 0, 0, 0, 0, 0, 0, 0, 0, 0, 0, 0, 0, 0, 0, 0, 0, 0, 0, 0, 0, 0, 0, 0, 0, 0, 0, 0, 0, 0, 0, 0, 0, 0, 0, 0, 0, 0, 0, 0, 0, 0, 0, 0, 0, 0, 0, 0, 0, 0, 0, 0, 0, 0, 0, 0, 0, 0, 0, 0, 0, 0, 0, 0, 0, 0, 0, 0, 0, 0, 0, 0, 0, 0, 0, 0, 0, 0, 0, 0, 0, 0, 0, 0, 0, 0, 0, 0, 0, 0, 0, 0, 0, 0, 0, 0, 0, 0, 0, 0, 0, 0, 0, 0, 0, 0, 0, 0, 0, 0, 0, 0, 0, 0, 0, 0, 0, 0, 0, 0, 0, 0, 0, 0, 0, 0, 0, 0, 0, 0, 0, 0, 0, 0, 0, 0, 0, 0, 0, 0, 0, 0, 0, 0, 0, 0, 0, 0, 0, 0, 0, 0, 0, 0, 0, 0, 0, 0, 0, 0, 0, 0, 0, 0, 0, 0, 0, 0, 0, 0, 0, 0, 0, 0, 0, 0, 0, 0, 0, 0, 0, 0, 0, 0, 0, 0, 0, 0, 0, 0, 0, 0, 0, 0, 0, 0, 0, 0, 0, 0, 0, 0, 0, 0, 0, 0, 0, 0, 0, 0, 0, 0, 0, 0, 0, 0, 0, 0, 0, 0, 0, 0, 0, 0, 0, 0, 0, 0, 0, 0, 0, 0, 0, 0, 0, 0, 0, 0, 0, 0, 0, 0, 0, 0, 0, 0, 0, 0, 0, 0, 0, 0, 0, 0, 0, 0, 0, 0, 0, 0, 0, 0, 0, 0, 0, 0, 0, 0, 0, 0, 0, 0, 0, 0, 0, 0, 0, 0, 0, 0, 0, 0, 0, 0, 0, 0, 0, 0, 0, 0, 0, 0, 0, 0, 0, 0, 0, 0, 0, 0, 0, 0, 0, 0, 0, 0, 0, 0, 0, 0, 0, 0, 0, 0, 0, 0, 0, 0, 0, 0, 0, 0, 0, 0, 0, 0, 0, 0, 0, 0, 0, 0, 0, 0, 0, 0, 0, 0, 0, 0, 0, 0, 0, 0, 0, 0, 0, 0, 0, 0, 0, 0, 0, 0, 0, 0, 0, 0, 0, 0, 0, 0, 0, 0, 0, 0, 0, 0, 0, 0, 0, 0, 0, 0, 0, 0, 0, 0, 0, 0, 0, 0, 0, 0, 0, 0, 0, 0, 0, 0, 0, 0, 0, 0, 0, 0, 0, 0, 0, 0, 0, 0, 0, 0, 0, 0, 0, 0, 0, 0, 0, 0, 0, 0, 0, 0, 0, 0, 0, 0, 0, 0, 0, 0, 0, 0, 0, 0, 0, 0, 0, 0, 0, 0, 0, 0, 0, 0, 0, 0, 0, 0, 0, 0, 0, 0, 0, 0, 0, 0, 0, 0, 0, 0, 0, 0, 0, 0, 0, 0, 0, 0, 0, 0, 0, 0, 0, 0, 0, 0, 0, 0, 0, 0, 0, 0, 0, 0, 0, 0, 0, 0, 0, 0, 0, 0, 0, 0, 0, 0, 0, 0, 0, 0, 0, 0, 0, 0, 0, 0, 0, 0, 0, 0, 0, 0, 0, 0, 0, 0, 0, 0, 0, 0, 0, 0, 0, 0, 0, 0, 0, 0, 0, 0, 0, 0, 0, 0, 0, 0, 0, 0, 0, 0, 0, 0, 0, 0, 0, 0, 0, 0, 0, 0, 0, 0, 0, 0, 0, 0, 0, 0, 0, 0, 0, 0, 0, 0, 0], "Pkt Loss Calc elements.Counter"=u32 0, "Pkt Loss Calc elements.En Calc"=TRUE) -> (w70:T1)
          }
          event User Event {
            w75 = -1  # The timeout case no longer executes
            # "This module called the \"Private.Stop Pkt Loss Calc\" private request."
            n367 = event-data() -> ()  [unwired: 1 in, 1 out]
            n368 = Bundle By Name(cluster=w73, "Pkt Loss Calc elements.En Calc"=FALSE) -> (w72:T1)
          }
          event User Event {
            # "This module called the \"Private.Update Packet ID\" private request."
            n369 = event-data() -> ("Packet ID"=w78:u32)  [unwired: 1 in]
            n370 = Unbundle By Name(w81) -> ("Pkt Loss Calc elements.Counter"=w79:u32, "Pkt Loss Calc elements.Array"=w80:u32[], "Pkt Loss Calc elements.En Calc"=w76:bool)
            n371 = case shown="True" w76 {
              tunnel: w81 -> [w83 w92]
              tunnel: w80 -> [_ w91]
              tunnel: w79 -> [_ w90]
              tunnel: w78 -> [_ w89]
              tunnel: [w83 w88] -> w77
              frame False {
                # "Ignore Incoming Pkt"
              }
              frame True {
                n372 = Replace Array Subset(array=w91, new element=w89, index=w90) -> (w84:u32[])
                n373 = Increment(x=w90) -> (x+1=w86:u32)
                n374 = Greater Or Equal?(x=w86, y=u32 1249) -> (x >= y?=w87:bool)
                n375 = Bundle By Name(cluster=w92, "Pkt Loss Calc elements.Counter"=w86, "Pkt Loss Calc elements.Array"=w84) -> (w88:T1)
                n376 = case shown="True" w87 {
                  tunnel: w84 -> [_ w93]
                  frame False {
                  }
                  frame True {
                    n377 = call "Calculate Packet Loss.vi"("Data Array"=w93) -> ()  [unwired: 10 in, 1 out]
                  }
                }
              }
            }
          }
          event User Event {
            # "Send to UI Module"
            # "Reinitialize all Calcs"
            # "This module called the \"Private.Calculate Packet Loss\" private request."
            n378 = event-data() -> ("Data Array"=w103:u32[])  [unwired: 1 in]
            n379 = call-poly <userlib>:"MGI Calculate Array Differences.vi"("x(i)"=w103) -> ("y(i)=x(i)-x(i-1)"=w102:dbl[])  [unwired: 1 in]
            n380 = Array Subset(array=w102, index=25, length=1200) -> (w99:dbl[])
            n381 = Add Array Elements(numeric array=w99) -> (sum=w95:dbl)
            n382 = Subtract(x=w95, y=1200.0) -> (x-y=w97:dbl)
            n383 = Divide(x=w97, y=12.0) -> (x/y=w94:dbl)
            n384 = call "Update Packet Loss (%).vi"("Paket Loss"=w94) -> ()  [unwired: 10 in, 1 out]
            n385 = Bundle By Name(cluster=w105, "Pkt Loss Calc elements.Array"=u32[] [0, 0, 0, 0, 0, 0, 0, 0, 0, 0, 0, 0, 0, 0, 0, 0, 0, 0, 0, 0, 0, 0, 0, 0, 0, 0, 0, 0, 0, 0, 0, 0, 0, 0, 0, 0, 0, 0, 0, 0, 0, 0, 0, 0, 0, 0, 0, 0, 0, 0, 0, 0, 0, 0, 0, 0, 0, 0, 0, 0, 0, 0, 0, 0, 0, 0, 0, 0, 0, 0, 0, 0, 0, 0, 0, 0, 0, 0, 0, 0, 0, 0, 0, 0, 0, 0, 0, 0, 0, 0, 0, 0, 0, 0, 0, 0, 0, 0, 0, 0, 0, 0, 0, 0, 0, 0, 0, 0, 0, 0, 0, 0, 0, 0, 0, 0, 0, 0, 0, 0, 0, 0, 0, 0, 0, 0, 0, 0, 0, 0, 0, 0, 0, 0, 0, 0, 0, 0, 0, 0, 0, 0, 0, 0, 0, 0, 0, 0, 0, 0, 0, 0, 0, 0, 0, 0, 0, 0, 0, 0, 0, 0, 0, 0, 0, 0, 0, 0, 0, 0, 0, 0, 0, 0, 0, 0, 0, 0, 0, 0, 0, 0, 0, 0, 0, 0, 0, 0, 0, 0, 0, 0, 0, 0, 0, 0, 0, 0, 0, 0, 0, 0, 0, 0, 0, 0, 0, 0, 0, 0, 0, 0, 0, 0, 0, 0, 0, 0, 0, 0, 0, 0, 0, 0, 0, 0, 0, 0, 0, 0, 0, 0, 0, 0, 0, 0, 0, 0, 0, 0, 0, 0, 0, 0, 0, 0, 0, 0, 0, 0, 0, 0, 0, 0, 0, 0, 0, 0, 0, 0, 0, 0, 0, 0, 0, 0, 0, 0, 0, 0, 0, 0, 0, 0, 0, 0, 0, 0, 0, 0, 0, 0, 0, 0, 0, 0, 0, 0, 0, 0, 0, 0, 0, 0, 0, 0, 0, 0, 0, 0, 0, 0, 0, 0, 0, 0, 0, 0, 0, 0, 0, 0, 0, 0, 0, 0, 0, 0, 0, 0, 0, 0, 0, 0, 0, 0, 0, 0, 0, 0, 0, 0, 0, 0, 0, 0, 0, 0, 0, 0, 0, 0, 0, 0, 0, 0, 0, 0, 0, 0, 0, 0, 0, 0, 0, 0, 0, 0, 0, 0, 0, 0, 0, 0, 0, 0, 0, 0, 0, 0, 0, 0, 0, 0, 0, 0, 0, 0, 0, 0, 0, 0, 0, 0, 0, 0, 0, 0, 0, 0, 0, 0, 0, 0, 0, 0, 0, 0, 0, 0, 0, 0, 0, 0, 0, 0, 0, 0, 0, 0, 0, 0, 0, 0, 0, 0, 0, 0, 0, 0, 0, 0, 0, 0, 0, 0, 0, 0, 0, 0, 0, 0, 0, 0, 0, 0, 0, 0, 0, 0, 0, 0, 0, 0, 0, 0, 0, 0, 0, 0, 0, 0, 0, 0, 0, 0, 0, 0, 0, 0, 0, 0, 0, 0, 0, 0, 0, 0, 0, 0, 0, 0, 0, 0, 0, 0, 0, 0, 0, 0, 0, 0, 0, 0, 0, 0, 0, 0, 0, 0, 0, 0, 0, 0, 0, 0, 0, 0, 0, 0, 0, 0, 0, 0, 0, 0, 0, 0, 0, 0, 0, 0, 0, 0, 0, 0, 0, 0, 0, 0, 0, 0, 0, 0, 0, 0, 0, 0, 0, 0, 0, 0, 0, 0, 0, 0, 0, 0, 0, 0, 0, 0, 0, 0, 0, 0, 0, 0, 0, 0, 0, 0, 0, 0, 0, 0, 0, 0, 0, 0, 0, 0, 0, 0, 0, 0, 0, 0, 0, 0, 0, 0, 0, 0, 0, 0, 0, 0, 0, 0, 0, 0, 0, 0, 0, 0, 0, 0, 0, 0, 0, 0, 0, 0, 0, 0, 0, 0, 0, 0, 0, 0, 0, 0, 0, 0, 0, 0, 0, 0, 0, 0, 0, 0, 0, 0, 0, 0, 0, 0, 0, 0, 0, 0, 0, 0, 0, 0, 0, 0, 0, 0, 0, 0, 0, 0, 0, 0, 0, 0, 0, 0, 0, 0, 0, 0, 0, 0, 0, 0, 0, 0, 0, 0, 0, 0, 0, 0, 0, 0, 0, 0, 0, 0, 0, 0, 0, 0, 0, 0, 0, 0, 0, 0, 0, 0, 0, 0, 0, 0, 0, 0, 0, 0, 0, 0, 0, 0, 0, 0, 0, 0, 0, 0, 0, 0, 0, 0, 0, 0, 0, 0, 0, 0, 0, 0, 0, 0, 0, 0, 0, 0, 0, 0, 0, 0, 0, 0, 0, 0, 0, 0, 0, 0, 0, 0, 0, 0, 0, 0, 0, 0, 0, 0, 0, 0, 0, 0, 0, 0, 0, 0, 0, 0, 0, 0, 0, 0, 0, 0, 0, 0, 0, 0, 0, 0, 0, 0, 0, 0, 0, 0, 0, 0, 0, 0, 0, 0, 0, 0, 0, 0, 0, 0, 0, 0, 0, 0, 0, 0, 0, 0, 0, 0, 0, 0, 0, 0, 0, 0, 0, 0, 0, 0, 0, 0, 0, 0, 0, 0, 0, 0, 0, 0, 0, 0, 0, 0, 0, 0, 0, 0, 0, 0, 0, 0, 0, 0, 0, 0, 0, 0, 0, 0, 0, 0, 0, 0, 0, 0, 0, 0, 0, 0, 0, 0, 0, 0, 0, 0, 0, 0, 0, 0, 0, 0, 0, 0, 0, 0, 0, 0, 0, 0, 0, 0, 0, 0, 0, 0, 0, 0, 0, 0, 0, 0, 0, 0, 0, 0, 0, 0, 0, 0, 0, 0, 0, 0, 0, 0, 0, 0, 0, 0, 0, 0, 0, 0, 0, 0, 0, 0, 0, 0, 0, 0, 0, 0, 0, 0, 0, 0, 0, 0, 0, 0, 0, 0, 0, 0, 0, 0, 0, 0, 0, 0, 0, 0, 0, 0, 0, 0, 0, 0, 0, 0, 0, 0, 0, 0, 0, 0, 0, 0, 0, 0, 0, 0, 0, 0, 0, 0, 0, 0, 0, 0, 0, 0, 0, 0, 0, 0, 0, 0, 0, 0, 0, 0, 0, 0, 0, 0, 0, 0, 0, 0, 0, 0, 0, 0, 0, 0, 0, 0, 0, 0, 0, 0, 0, 0, 0, 0, 0, 0, 0, 0, 0, 0, 0, 0, 0, 0, 0, 0, 0, 0, 0, 0, 0, 0, 0, 0, 0, 0, 0, 0, 0, 0, 0, 0, 0, 0, 0, 0, 0, 0, 0, 0, 0, 0, 0, 0, 0, 0, 0, 0, 0, 0, 0, 0, 0, 0, 0, 0, 0, 0, 0, 0, 0, 0, 0, 0, 0, 0, 0, 0, 0, 0, 0, 0, 0, 0, 0, 0, 0, 0, 0, 0, 0, 0, 0, 0, 0, 0, 0, 0, 0, 0, 0, 0, 0, 0, 0, 0, 0, 0, 0, 0, 0, 0, 0, 0, 0, 0, 0, 0, 0, 0, 0, 0, 0, 0, 0, 0, 0, 0, 0, 0, 0, 0, 0, 0, 0, 0, 0, 0, 0, 0, 0, 0, 0, 0, 0, 0, 0, 0, 0, 0, 0, 0, 0, 0, 0, 0, 0, 0, 0, 0, 0, 0, 0, 0, 0, 0, 0, 0, 0, 0, 0, 0, 0, 0, 0, 0, 0, 0, 0, 0, 0, 0, 0, 0, 0, 0, 0, 0, 0, 0, 0, 0, 0, 0, 0, 0, 0, 0, 0, 0, 0, 0, 0, 0, 0, 0, 0, 0, 0, 0, 0, 0, 0, 0, 0, 0, 0, 0, 0, 0, 0, 0, 0, 0, 0, 0, 0, 0, 0, 0, 0, 0, 0, 0, 0, 0, 0, 0, 0, 0, 0, 0, 0, 0, 0, 0, 0, 0, 0, 0, 0, 0, 0, 0, 0, 0, 0, 0, 0, 0, 0, 0, 0, 0, 0, 0, 0, 0, 0, 0, 0, 0, 0, 0, 0, 0, 0, 0, 0, 0, 0, 0], "Pkt Loss Calc elements.Counter"=u32 0) -> (w104:T1)
          }
        }
        n386 = call-dynamic "Delacor_lib_QMH_Error Handler - Helper Loop.vi"("Error Debug"=w52, "error in"=w54, "Message Queue in"=w53) -> ()  [unwired: 7 in, 2 out]
      }
      n387 = Unregister For Events(event registration refnum=w36) -> ()  [unwired: 1 in, 1 out]
    }
    frame Error {
      # "Synchronize Caller Events.vi will inform Start Module.vi that the module has launched and will let the code calling Start Module.vi register for broadcasts and would permit the caller receive the broadcast that an error occurred at launch time."
      n388 = call "Synchronize Caller Events.vi"("Singleton Module Admin in"=w932) -> ("error out"=w937:errorcluster)  [unwired: 9 in, 1 out]
      n389 = call-dynamic "Delacor_lib_QMH_Release Message Queue.vi"("error in"=w928, "Message Queue"=w929) -> ("error out"=w927:errorcluster)  [unwired: 9 in]
      n390 = call "Module Name--constant.vi"() -> ("Module Name"=w935:string)  [unwired: 11 in]
      n391 = case "Settings Editor was\nalready running?" shown="False" w930 {
        frame False {
          n392 = call "Module Name--constant.vi"() -> ("Module Name"=w940:string)  [unwired: 11 in]
          n393 = call "Stop Module.vi"("Wait for Module to Stop? (F)"=TRUE, "Origin"=w940) -> ()  [unwired: 9 in, 1 out]
        }
        frame True {
          # "Another Module is\nin charge of stopping Settings Editor"
        }
      }
      n394 = Format Into String(format string="An error occurred during initialization. %s is no longer running.", w935) -> (resulting string=w933:string)  [unwired: 2 in, 1 out]
      n395 = Merge Errors(w927, w937) -> (w938:errorcluster)
      n396 = call "Error Reported.vi"("Additional Information"=w933, "Error"=w938) -> ()  [unwired: 9 in, 1 out]
    }
  }
  n397 = Merge Errors(w30, w32) -> (w29:errorcluster)
  n398 = call "Close Module.vi"("error in (no error)"=w29, "Module Admin in"=w19) -> ("error out"=w22:errorcluster, "External Launch"=w13:bool, "Module Admin out"=w14:refnum<class "Delacor_lib_QMH_Module Admin.lvclass">)  [unwired: 7 in]
  n399 = Unregister For Events(event registration refnum=w4, error in=w22) -> (error out=w20:errorcluster)
  n400 = Unregister For Events(event registration refnum=w18, error in=w22) -> (error out=w28:errorcluster)
  n401 = case "External Launch?" shown="True" w13 {
    tunnel: w28 -> [_ w941]
    frame False {
    }
    frame True {
      n402 = case shown="No Error" w941 {
        frame No Error {
          n403 = invoke class="VI" method="FP.Close"() -> ()  [unwired: 3 in, 3 out]
        }
        frame Error {
          n404 = invoke class="VI" method="FP.Open"("Activate"=TRUE ("Activate?")) -> ()  [unwired: 4 in, 5 out]
        }
      }
    }
  }
  n405 = local write "Module Admin"(w14) -> ()
  n406 = Merge Errors(w28, w20) -> (→"error out":errorcluster)
